vi "-Autonomous Independent.vi"() -> ()   [LabVIEW 2012]
doc: "This VI is called when autonomous begins, and will automatically be terminated when autonomous ends. You can carry out timed or sensor driven robot movement independently without needing to return to the caller."
uses:
  <vilib>/Rock Robotics/WPI/Solenoid/WPI_SolenoidValue.ctl
  Robot Global Data.vi
  <vilib>/Rock Robotics/WPI/RobotDrive/WPI_RobotDriveGetSetRefNum.vi
  <vilib>/addons/control/pid/pid.llb/PID (DBL).vi
  <vilib>/Rock Robotics/WPI/Joystick/WPI_JoystickGetSetRefNum.vi
  <vilib>/Rock Robotics/WPI/Solenoid/WPI_SolenoidSetEnum.vi
  <vilib>/addons/control/pid/NI_PID_pid.lvlib
panel:
  out "Field Position":T1(ring)
  in  "PID gains":T2={"proportional gain (Kc)"=1.0, "integral time (Ti, min)"=0.01, "derivative time (Td, min)"=0.0} {"derivative time (Td, min)" format="%.3f"; "integral time (Ti, min)" format="%.3f"; "proportional gain (Kc)" format="%.3f"}
  in  "Sweet Spot":dbl
  out "tick":dbl
  in  "wait time":dbl
  in  "Fast-Slow Variable":dbl=2.0
  out "Numeric 0":dbl
  out "Current Movement, for debugging":T3 {"Y Joystick Value" scale=1.0..-1.0; "X Joystick Value" scale=-1.0..1.0}
  in  "Array of robot movements":T4(array[cluster]) {"Y Joystick Value" scale=1.0..-1.0; "X Joystick Value" scale=-1.0..1.0}
  # "Be sure to right-click and choose Data Operations>>Make Current Value default if you want to save the array values with the VI"
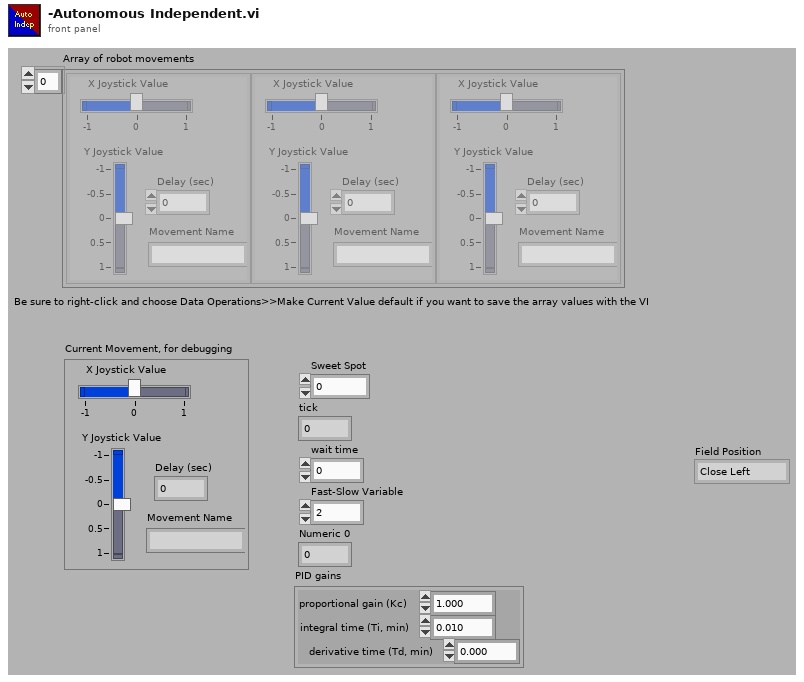
[diagram p1: front panel]
types:
  T1 = enum16{"Close Left", "Close Right", "Far Left", "Far Right"}
  T2 = cluster{"proportional gain (Kc)":dbl, "integral time (Ti, min)":dbl, "derivative time (Td, min)":dbl}
  T3 = cluster{"X Joystick Value":dbl, "Y Joystick Value":dbl, "Delay (sec)":dbl, "Movement Name":string}
  T4 = cluster{"X Joystick Value":dbl, "Y Joystick Value":dbl, "Delay (sec)":dbl, "Movement Name":string}[]
  T5 = typedef "WPI_JoystickDevRef.ctl" = cluster{"Device":T6}
  T6 = typedef "WPI_JoystickDeviceEnum.ctl" = enum16{"USB 1", "USB 2", "USB 3", "USB 4", "Kinect 1", "Kinect 2"}
  T7 = cluster{"axis 1 (x)":dbl, "axis 2 (y)":dbl, "axis 3 (throttle)":dbl, "axis 4":dbl, "axis 5":dbl, "axis 6":dbl}
  T8 = typedef "WPI_SolenoidValue.ctl" = enum16{"Off", "On", "Forward", "Reverse"}
  T9 = typedef "WPI_RobotDriveDevRef.ctl" = cluster{"DevStatus":errorcluster, "Motors[]":T10[], "Square Inputs":bool, "Max Output":dbl, "Isochronous":bool}
  T10 = typedef "WPI_MotorControlDeviceRef.ctl" = cluster{"DeviceStatus":errorcluster, "Type":enum16{"PWM", "CAN"}, "PWM":cluster{"Digital Module":T11, "PWM Channel":T12, "DeadBand":T13}, "CAN":cluster{"Device Number":u8, "Control Mode":T14, "Semaphore":T15, "Max Vout":dbl}, "Invert":bool, "TransformRef":T16, "InvTransformRef":T16}
  T11 = typedef "FPGA_TypedefDigitalModule.ctl" = enum16{"Digital Module 1", "Digital Module 2"}
  T12 = typedef "FPGA_DIOPWMChannel.ctl" = enum8{"PWM 1", "PWM 2", "PWM 3", "PWM 4", "PWM 5", "PWM 6", "PWM 7", "PWM 8", "PWM 9", "PWM 10", "Invalid"}
  T13 = typedef "WPI_PWMDeadband.ctl" = cluster{"Name":string, "maxPositivePwm":i32, "minPositivePwm":i32, "centerPwm":i32, "maxNegativePwm":i32, "minNegativePwm":i32, "angularRange":u16}
  T14 = typedef "WPI_CANJaguar_ControlMode.ctl" = enum8{"Percent VBus", "Current", "Speed", "Position", "Voltage"}
  T15 = typedef "Semaphore RefNum" = refnum<k1>
  T16 = typedef "WPI_PWMTransform_ConPane.ctl" = refnum<vi>
  T17 = cluster{"Center Position":cluster{"X":dbl, "Y":dbl}, "Distance (ft)":dbl, "Center":bool}[]
  T18 = cluster{"Target Info[0]":cluster{"Center Position":cluster{"X":dbl, "Y":dbl}, "Distance (ft)":dbl, "Center":bool}, "Target Info[1]":cluster{"Center Position":cluster{"X":dbl, "Y":dbl}, "Distance (ft)":dbl, "Center":bool}, "Target Info[2]":cluster{"Center Position":cluster{"X":dbl, "Y":dbl}, "Distance (ft)":dbl, "Center":bool}, "Target Info[3]":cluster{"Center Position":cluster{"X":dbl, "Y":dbl}, "Distance (ft)":dbl, "Center":bool}, "Target Info[4]":cluster{"Center Position":cluster{"X":dbl, "Y":dbl}, "Distance (ft)":dbl, "Center":bool}, "Target Info[5]":cluster{"Center Position":cluster{"X":dbl, "Y":dbl}, "Distance (ft)":dbl, "Center":bool}, "Target Info[6]":cluster{"Center Position":cluster{"X":dbl, "Y":dbl}, "Distance (ft)":dbl, "Center":bool}, "Target Info[7]":cluster{"Center Position":cluster{"X":dbl, "Y":dbl}, "Distance (ft)":dbl, "Center":bool}, "Target Info[8]":cluster{"Center Position":cluster{"X":dbl, "Y":dbl}, "Distance (ft)":dbl, "Center":bool}}
  T19 = cluster{"Center Position":cluster{"X":dbl, "Y":dbl}, "Distance (ft)":dbl, "Center":bool}
  T20 = typedef "WPI_SolenoidDevRef.ctl" = cluster{"DevStatus":errorcluster, "Solenoid Module":T21, "Forward Solenoid Channel":T22, "Reverse Solenoid Channel":T22}
  T21 = typedef "FPGA_TypedefSolenoidModule.ctl" = enum16{"Solenoid Module 1", "Solenoid Module 2"}
  T22 = typedef "WPI_SolenoidChannel.ctl" = enum8{"Solenoid 1", "Solenoid 2", "Solenoid 3", "Solenoid 4", "Solenoid 5", "Solenoid 6", "Solenoid 7", "Solenoid 8", "Invalid"}
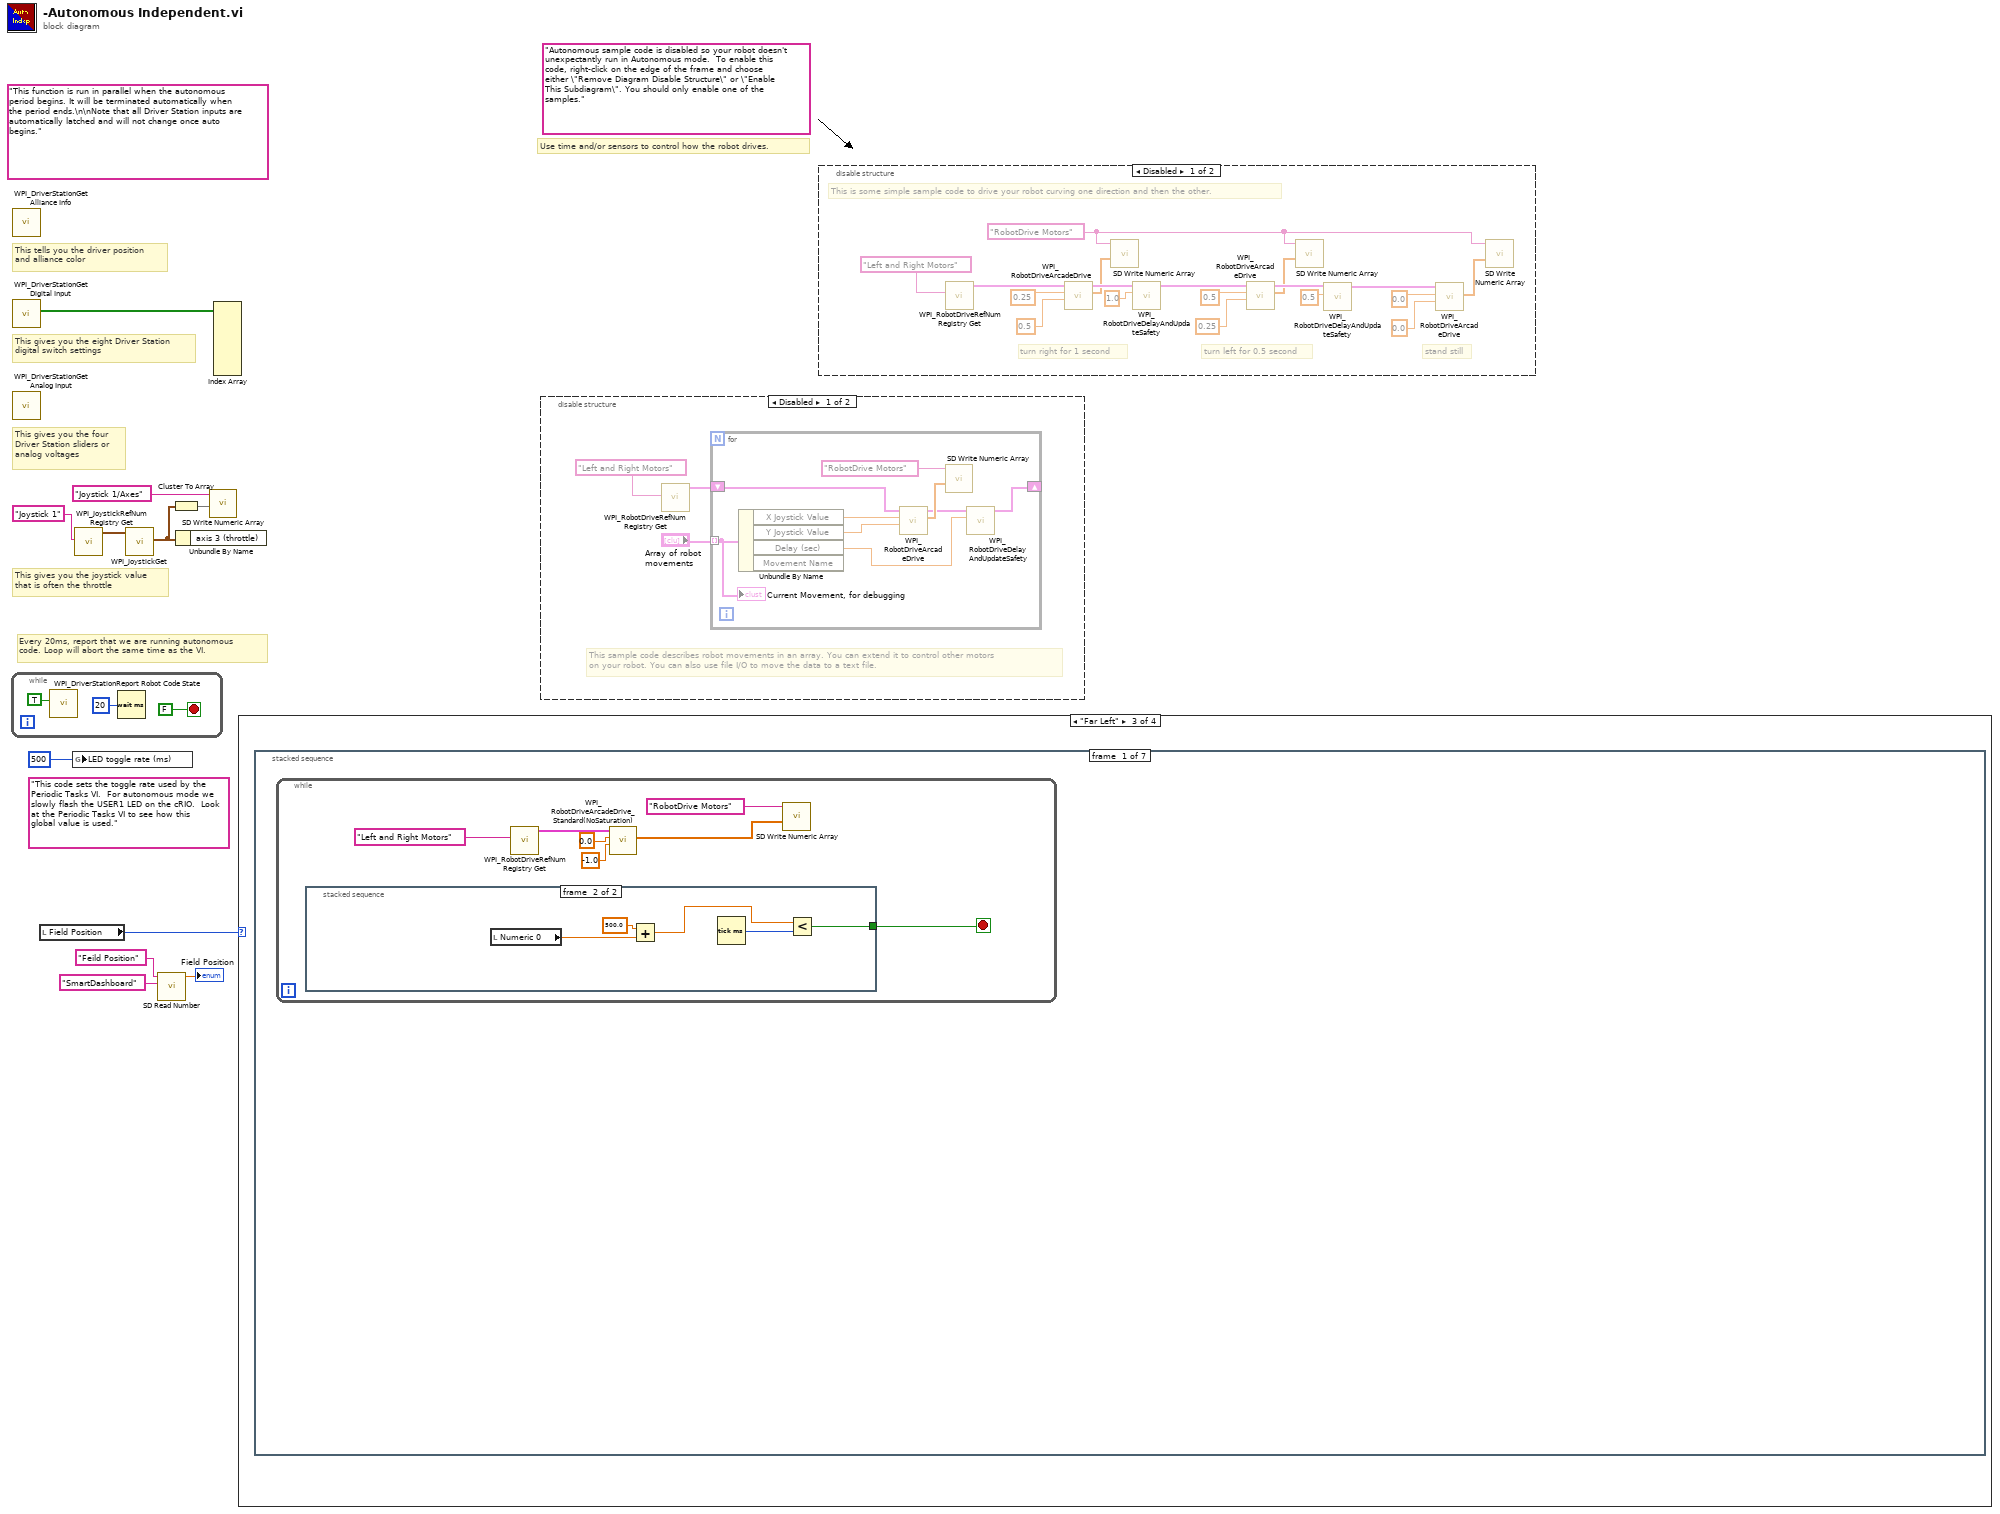
[diagram p0: block diagram]
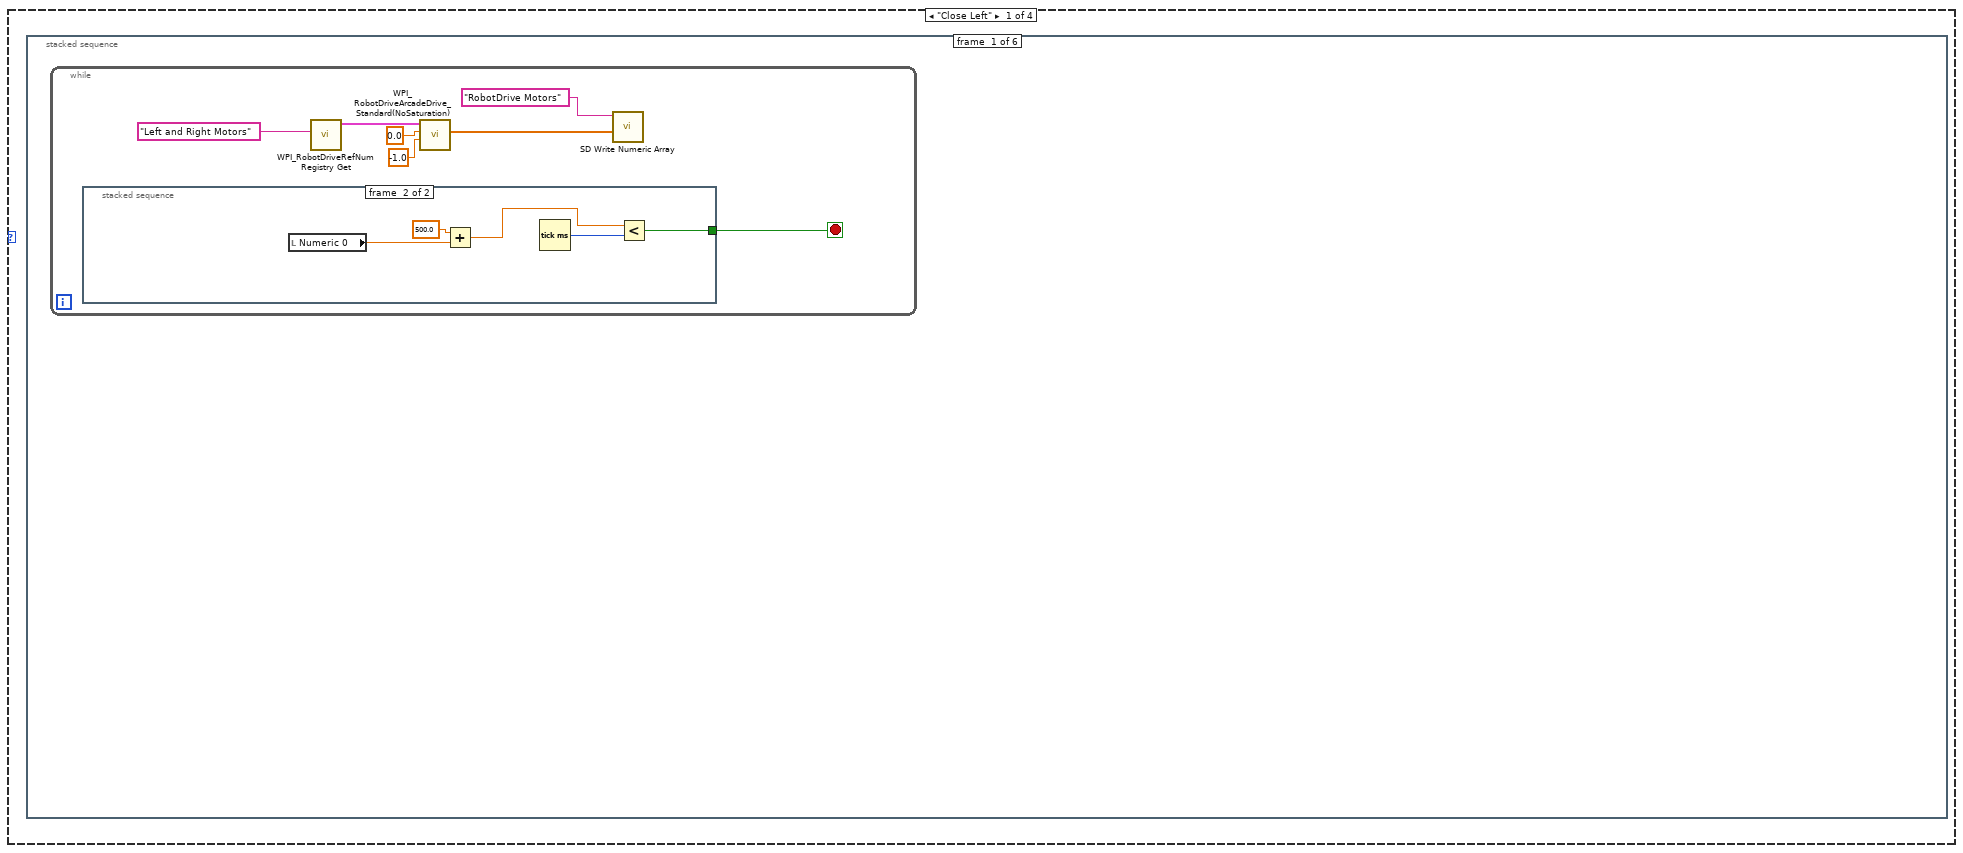
[diagram p2: hidden frame]
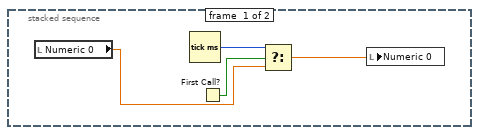
[diagram p3: hidden frame]
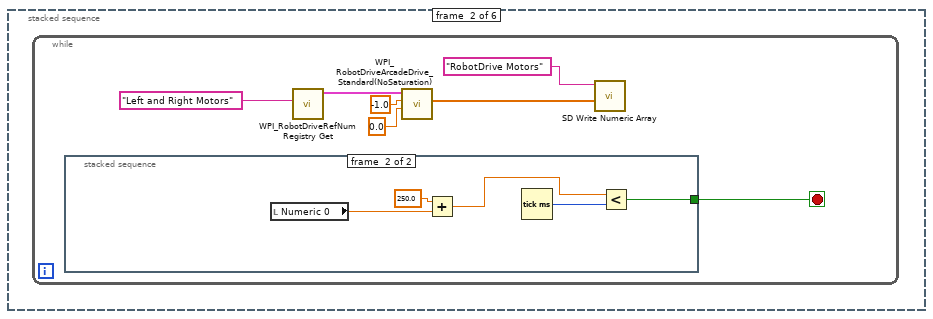
[diagram p4: hidden frame]
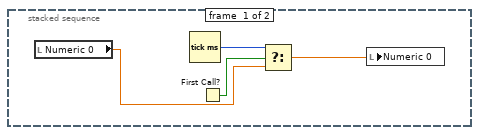
[diagram p5: hidden frame]
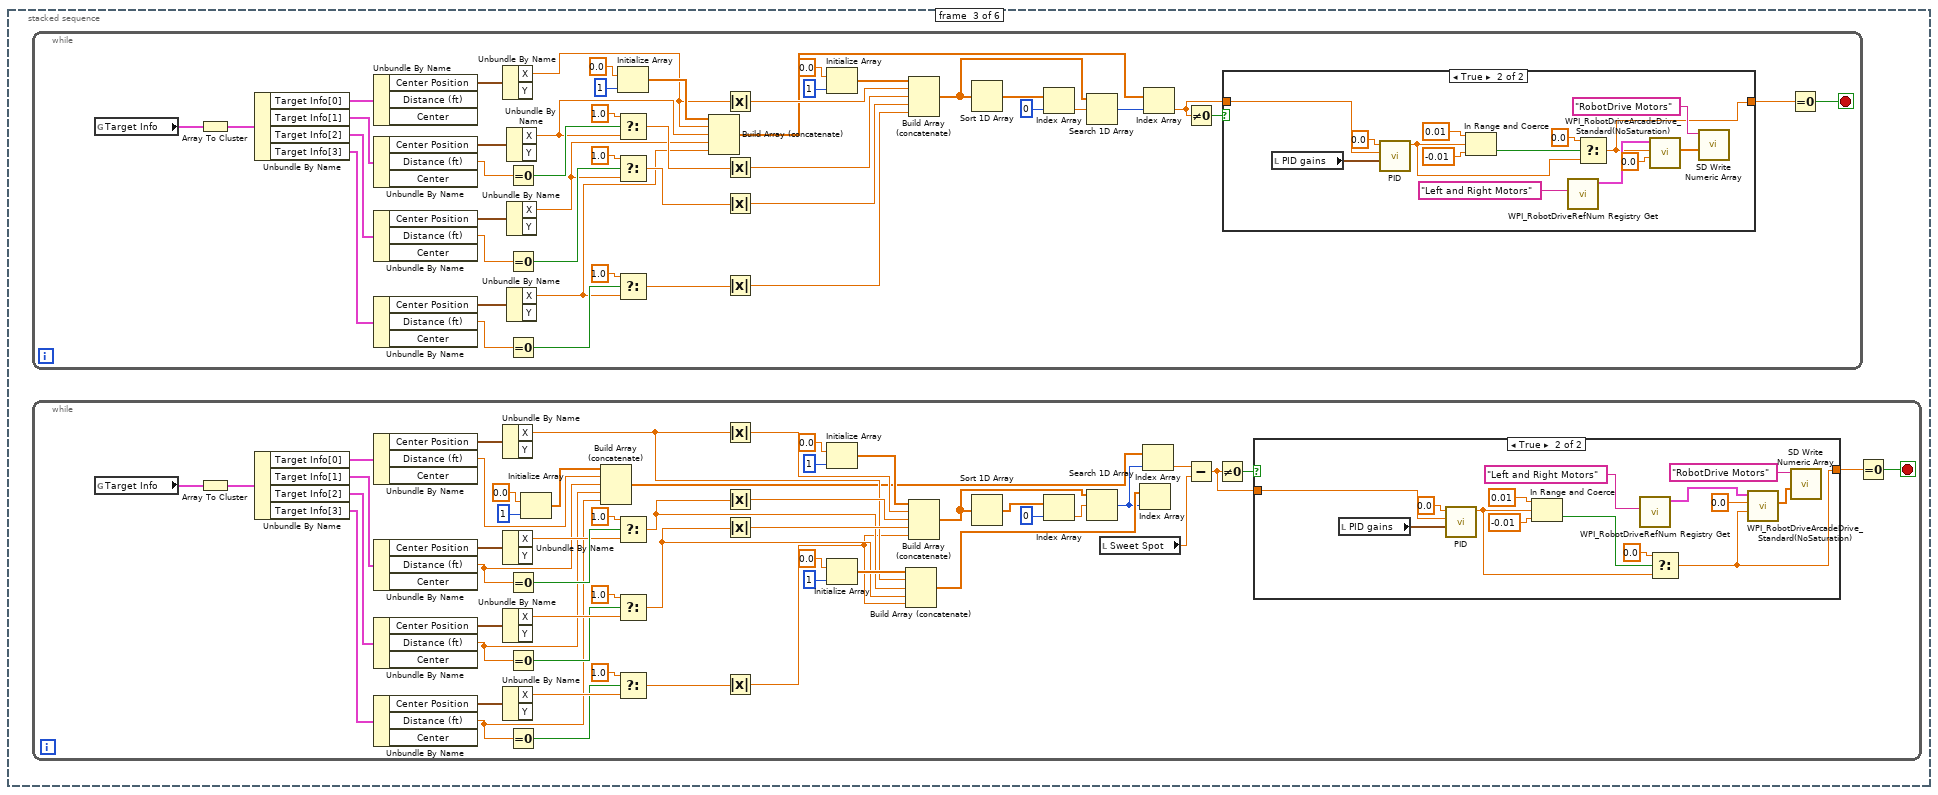
[diagram p6: hidden frame]
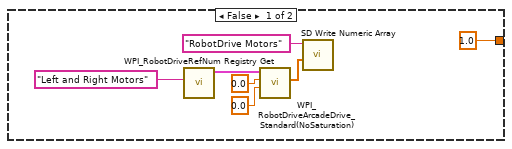
[diagram p7: hidden frame]
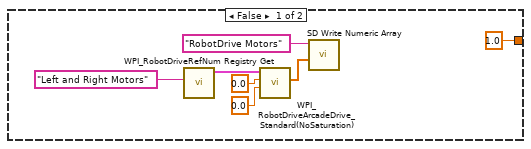
[diagram p8: hidden frame]
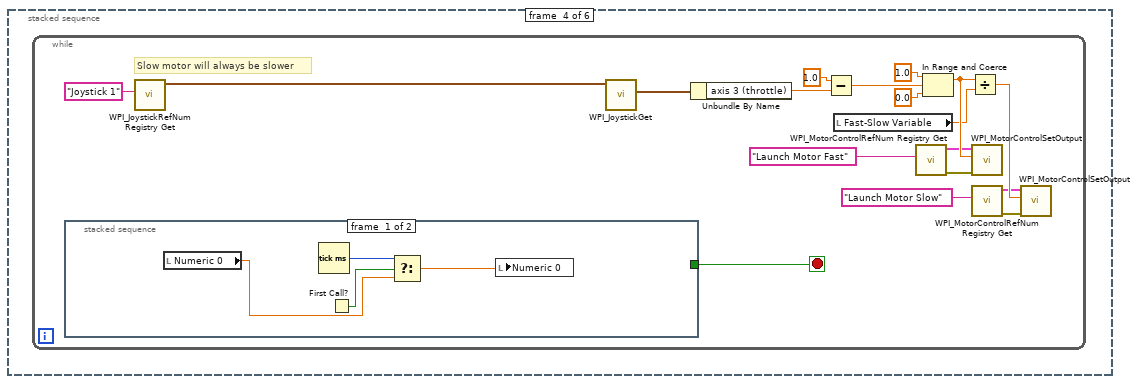
[diagram p9: hidden frame]
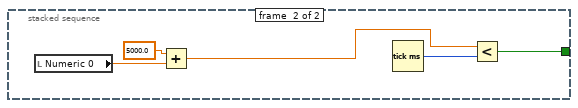
[diagram p10: hidden frame]
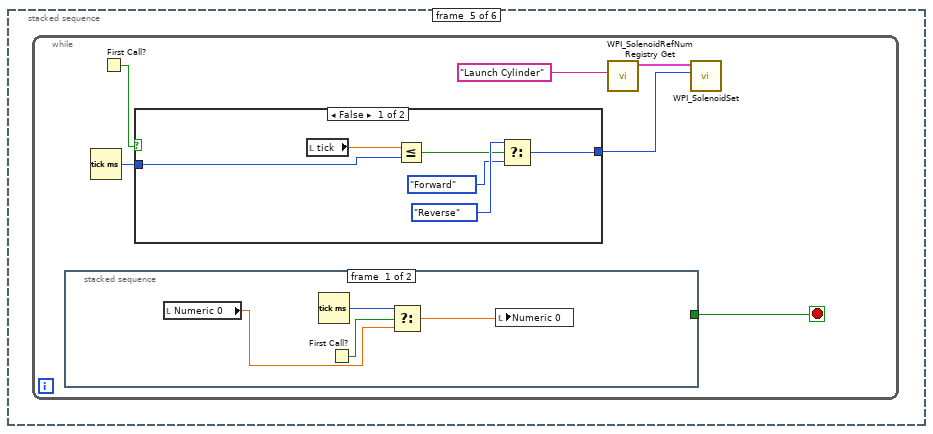
[diagram p11: hidden frame]
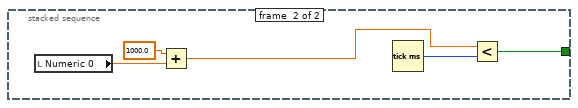
[diagram p12: hidden frame]
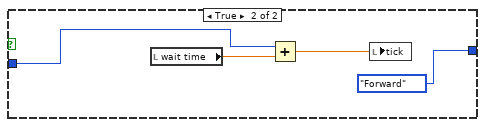
[diagram p13: hidden frame]
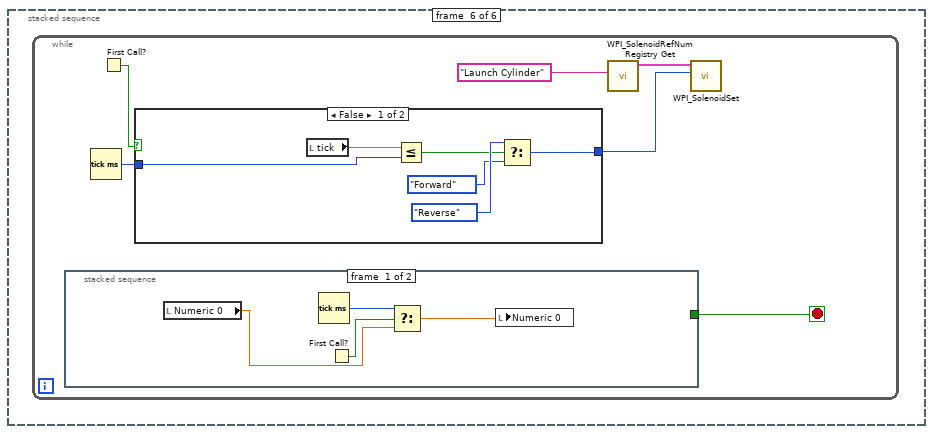
[diagram p14: hidden frame]
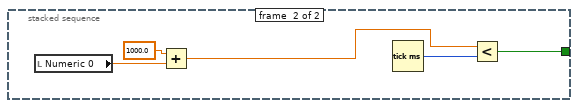
[diagram p15: hidden frame]
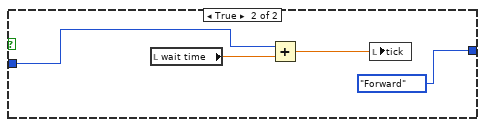
[diagram p16: hidden frame]
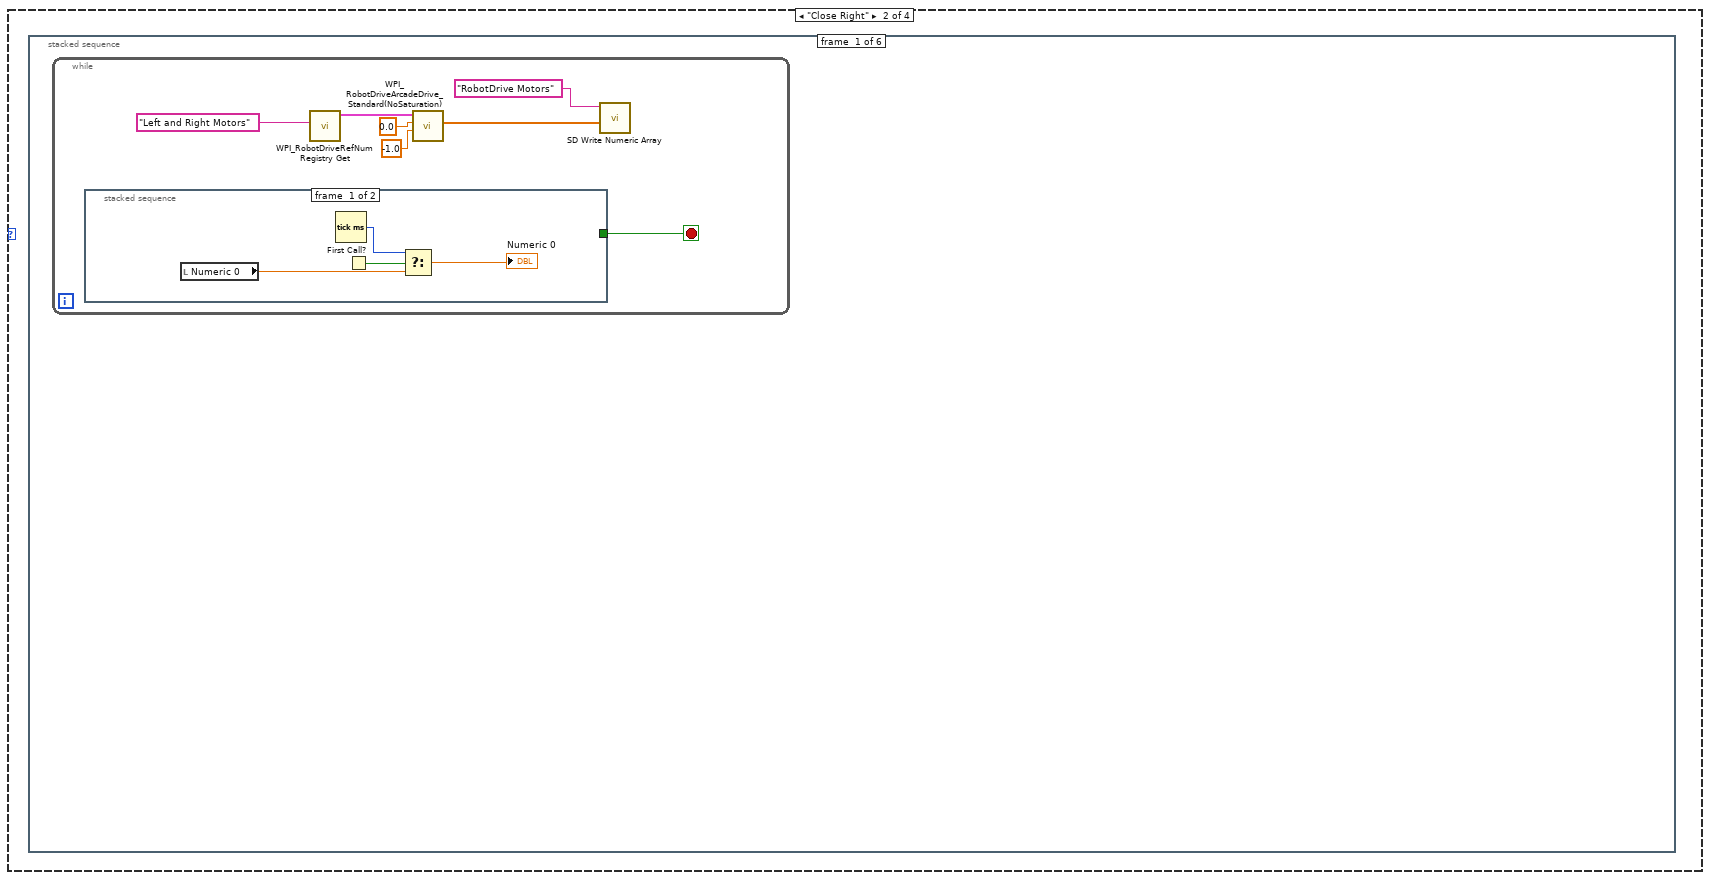
[diagram p17: hidden frame]
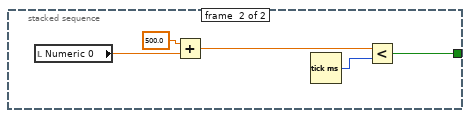
[diagram p18: hidden frame]
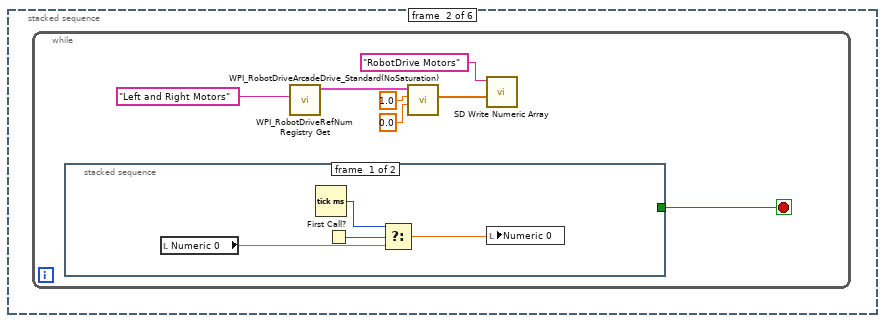
[diagram p19: hidden frame]
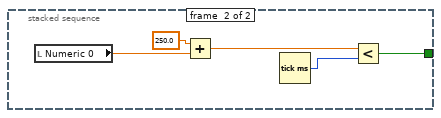
[diagram p20: hidden frame]
diagram:
  (unwired) "This code sets the toggle rate used by the Periodic Tasks VI.  For autonomous mode we slowly flash the USER1 LED on the cRIO.  Look at the Periodic Tasks VI to see how this global value is used."
  (unwired) "Autonomous sample code is disabled so your robot doesn't unexpectantly run in Autonomous mode.  To enable this code, right-click on the edge of the frame and choose either \"Remove Diagram Disable Structure\" or \"Enable This Subdiagram\". You should only enable one of the samples."
  (unwired) "This function is run in parallel when the autonomous period begins. It will be terminated automatically when the period ends.\n\nNote that all Driver Station inputs are automatically latched and will not change once auto begins."
  # "Every 20ms, report that we are running autonomous\ncode. Loop will abort the same time as the VI."
  # "This gives you the joystick value\nthat is often the throttle"
  # "Use time and/or sensors to control how the robot drives."
  # "This tells you the driver position\nand alliance color"
  # "This gives you the eight Driver Station\ndigital switch settings"
  # "This gives you the four\nDriver Station sliders or\nanalog voltages"
  n1 = while {
    stop <- FALSE stop-if-true
    n2 = call <vilib>:"WPI_DriverStationReport Robot Code State.vi"("Autonomous"=TRUE) -> ()  [unwired: 10 in, 1 out]
    n3 = Wait (ms)(milliseconds to wait=u32 20) -> ()  [unwired: 1 out]
  }
  n4 = call <vilib>:"WPI_DriverStationGet Alliance Info.vi"() -> ()  [unwired: 12 out]
  n5 = call <vilib>:"WPI_DriverStationGet Digital Input.vi"() -> ("Driver Station Digital Input (1-8)"=w11:bool[])  [unwired: 11 out]
  n6 = call <vilib>:"WPI_DriverStationGet Analog Input.vi"() -> ()  [unwired: 12 out]
  n7 = local read "Field Position"() -> (w1:T1)
  n8 = global write "Robot Global Data.vi" "LED toggle rate (ms)"(u32 500 ("LED ms toggle rate")) -> ()
  n9 = call <vilib>:"WPI_JoystickRefNum Registry Get.vi"("refnum name"="Joystick 1") -> ("JoystickDevRef"=w9:T5)  [unwired: 1 in, 9 out]
  n10 = call <vilib>:"WPI_JoystickGet.vi"("JoystickDevRef"=w9) -> ("Axes"=w6:T7)  [unwired: 1 in, 5 out]
  n11 = call <vilib>:"SD Read Number.vi"("Table Prefix"="SmartDashboard", "Name"="Feild Position") -> ("Numeric"=→"Field Position":dbl)  [unwired: 7 in, 2 out]
  n12 = Cluster To Array(cluster=w6) -> (array=w7:dbl[])
  n13 = Unbundle By Name(w6) -> ()  [unwired: 1 out]
  n14 = call <vilib>:"SD Write Numeric Array.vi"("Numeric Array"=w7, "Name"="Joystick 1/Axes") -> ()  [unwired: 8 in, 2 out]
  n15 = Index Array(array=w11) -> ()  [unwired: 8 in, 8 out]
  n16 = case shown="\"Far Left\"" w1 {
    frame "Close Left" {
      n17 = stacked-sequence {
        frame #0 {
          n18 = while {
            stop <- w15 stop-if-true
            n19 = stacked-sequence {
              tunnel: [_ w26] -> w15
              frame #0 {
                n20 = local read "Numeric 0"() -> (w23:dbl)
                n21 = Tick Count (ms)() -> (millisecond timer value=w24:u32)
                n22 = First Call?() -> (First Call?: T/F=w25:bool)
                n23 = Select(t=w24, s=w25, f=w23) -> (s? t:f=w22:dbl)
                n24 = local write "Numeric 0"(w22) -> ()
              }
              frame #1 {
                n25 = local read "Numeric 0"() -> (w29:dbl)
                n26 = Add(x=500.0, y=w29) -> (x+y=w28:dbl)
                n27 = Tick Count (ms)() -> (millisecond timer value=w27:u32)
                n28 = Less?(x=w28, y=w27) -> (x < y?=w26:bool)
              }
            }
            n29 = call <vilib>:"WPI_RobotDriveRefNum Registry Get.vi"("refnum name"="Left and Right Motors") -> ("RobotDriveDevRef"=w20:T9)  [unwired: 1 in, 9 out]
            n30 = call <vilib>:"WPI_RobotDriveArcadeDrive_Standard(NoSaturation).vi"("Y axis value"=-1.0 ("X axis value"), "X axis value"=0.0, "RobotDriveDevRef"=w20) -> ("Motor Values"=w18:dbl[])  [unwired: 1 in, 7 out]
            n31 = call <vilib>:"SD Write Numeric Array.vi"("Numeric Array"=w18, "Name"="RobotDrive Motors") -> ()  [unwired: 8 in, 2 out]
          }
        }
        frame #1 {
          n32 = while {
            stop <- w31 stop-if-true
            n33 = stacked-sequence {
              tunnel: [_ w42] -> w31
              frame #0 {
                n34 = local read "Numeric 0"() -> (w39:dbl)
                n35 = Tick Count (ms)() -> (millisecond timer value=w40:u32)
                n36 = First Call?() -> (First Call?: T/F=w41:bool)
                n37 = Select(t=w40, s=w41, f=w39) -> (s? t:f=w38:dbl)
                n38 = local write "Numeric 0"(w38) -> ()
              }
              frame #1 {
                n39 = local read "Numeric 0"() -> (w45:dbl)
                n40 = Add(x=250.0, y=w45) -> (x+y=w44:dbl)
                n41 = Tick Count (ms)() -> (millisecond timer value=w43:u32)
                n42 = Less?(x=w44, y=w43) -> (x < y?=w42:bool)
              }
            }
            n43 = call <vilib>:"WPI_RobotDriveRefNum Registry Get.vi"("refnum name"="Left and Right Motors") -> ("RobotDriveDevRef"=w33:T9)  [unwired: 1 in, 9 out]
            n44 = call <vilib>:"WPI_RobotDriveArcadeDrive_Standard(NoSaturation).vi"("Y axis value"=0.0 ("X axis value"), "X axis value"=-1.0, "RobotDriveDevRef"=w33) -> ("Motor Values"=w35:dbl[])  [unwired: 1 in, 7 out]
            n45 = call <vilib>:"SD Write Numeric Array.vi"("Numeric Array"=w35, "Name"="RobotDrive Motors") -> ()  [unwired: 8 in, 2 out]
          }
        }
        frame #2 {
          n46 = while {
            stop <- w74 stop-if-true
            n47 = global read "Robot Global Data.vi" "Target Info"() -> (w92:T17)
            n48 = Array To Cluster(array=w92) -> (cluster=w91:T18)
            n49 = Unbundle By Name(w91) -> ("Target Info[0]"=w90:T19, "Target Info[1]"=w85:T19, "Target Info[2]"=w84:T19, "Target Info[3]"=w83:T19)
            n50 = Unbundle By Name(w90) -> ("Center Position"=w89:cluster{"X":dbl, "Y":dbl})  [unwired: 2 out]
            n51 = Unbundle By Name(w85) -> ("Center Position"=w88:cluster{"X":dbl, "Y":dbl}, "Distance (ft)"=w51:dbl)  [unwired: 1 out]
            n52 = Unbundle By Name(w84) -> ("Center Position"=w87:cluster{"X":dbl, "Y":dbl}, "Distance (ft)"=w53:dbl)  [unwired: 1 out]
            n53 = Unbundle By Name(w83) -> ("Center Position"=w86:cluster{"X":dbl, "Y":dbl}, "Distance (ft)"=w55:dbl)  [unwired: 1 out]
            n54 = Unbundle By Name(w89) -> ("X"=w49:dbl)  [unwired: 1 out]
            n55 = Unbundle By Name(w88) -> ("X"=w50:dbl)  [unwired: 1 out]
            n56 = Unbundle By Name(w87) -> ("X"=w52:dbl)  [unwired: 1 out]
            n57 = Unbundle By Name(w86) -> ("X"=w54:dbl)  [unwired: 1 out]
            n58 = Equal To 0?(x=w51) -> (x = 0?=w82:bool)
            n59 = Equal To 0?(x=w53) -> (x = 0?=w81:bool)
            n60 = Equal To 0?(x=w55) -> (x = 0?=w80:bool)
            n61 = Initialize Array(0.0 ("element"), 1 ("dimension size")) -> (w58:dbl[])
            n62 = Select(t=1.0, s=w82, f=w50) -> (s? t:f=w63:dbl)
            n63 = Select(t=1.0, s=w81, f=w52) -> (s? t:f=w62:dbl)
            n64 = Select(t=1.0, s=w80, f=w54) -> (s? t:f=w76:dbl)
            n65 = Build Array (concatenate)(w58, w49, w50, w52, w54) -> (w57:dbl[])
            n66 = Absolute Value(x=w49) -> (abs(x)=w70:dbl)
            n67 = Absolute Value(x=w63) -> (abs(x)=w69:dbl)
            n68 = Absolute Value(x=w62) -> (abs(x)=w68:dbl)
            n69 = Absolute Value(x=w76) -> (abs(x)=w61:dbl)
            n70 = Initialize Array(0.0 ("element"), 1 ("dimension size")) -> (w71:dbl[])
            n71 = Build Array (concatenate)(w71, w70, w69, w68, w61) -> (w64:dbl[])
            n72 = Sort 1D Array(array=w64) -> (sorted array=w67:dbl[])
            n73 = Index Array(array=w67, index=0) -> (element=w65:dbl)
            n74 = Search 1D Array(1D array=w64, element=w65) -> (index of element=w56:i32)  [unwired: 1 in]
            n75 = Index Array(array=w57, index=w56) -> (element=w47:dbl)
            n76 = Not Equal To 0?(x=w47) -> (x != 0?=w48:bool)
            n77 = case shown="True" w48 {
              tunnel: [1.0 ("output") w102] -> w75
              tunnel: w47 -> [_ w101]
              frame False {
                n78 = call <vilib>:"WPI_RobotDriveRefNum Registry Get.vi"("refnum name"="Left and Right Motors") -> ("RobotDriveDevRef"=w98:T9)  [unwired: 1 in, 9 out]
                n79 = call <vilib>:"WPI_RobotDriveArcadeDrive_Standard(NoSaturation).vi"("Y axis value"=0.0, "X axis value"=0.0, "RobotDriveDevRef"=w98) -> ("Motor Values"=w96:dbl[])  [unwired: 1 in, 7 out]
                n80 = call <vilib>:"SD Write Numeric Array.vi"("Numeric Array"=w96, "Name"="RobotDrive Motors") -> ()  [unwired: 8 in, 2 out]
              }
              frame True {
                n81 = local read "PID gains"() -> (w100:T2)
                n82 = call-poly <vilib>:"PID.vi"("PID gains"=w100, "process variable"=w101, "setpoint"=0.0 ("process variable")) -> ("output"=w103:dbl)  [unwired: 7 in, 1 out]
                n83 = In Range and Coerce(upper limit=0.01, x=w103, lower limit=-0.01) -> (In Range?=w105:bool)  [unwired: 1 out]
                n84 = call <vilib>:"WPI_RobotDriveRefNum Registry Get.vi"("refnum name"="Left and Right Motors") -> ("RobotDriveDevRef"=w111:T9)  [unwired: 1 in, 9 out]
                n85 = Select(t=0.0, s=w105, f=w103) -> (s? t:f=w102:dbl)
                n86 = call <vilib>:"WPI_RobotDriveArcadeDrive_Standard(NoSaturation).vi"("Y axis value"=0.0, "X axis value"=w102, "RobotDriveDevRef"=w111) -> ("Motor Values"=w110:dbl[])  [unwired: 1 in, 7 out]
                n87 = call <vilib>:"SD Write Numeric Array.vi"("Numeric Array"=w110, "Name"="RobotDrive Motors") -> ()  [unwired: 8 in, 2 out]
              }
            }
            n88 = Equal To 0?(x=w75) -> (x = 0?=w74:bool)
          }
          n89 = while {
            stop <- w145 stop-if-true
            n90 = global read "Robot Global Data.vi" "Target Info"() -> (w166:T17)
            n91 = Array To Cluster(array=w166) -> (cluster=w165:T18)
            n92 = Unbundle By Name(w165) -> ("Target Info[0]"=w164:T19, "Target Info[1]"=w159:T19, "Target Info[2]"=w158:T19, "Target Info[3]"=w157:T19)
            n93 = Unbundle By Name(w164) -> ("Center Position"=w163:cluster{"X":dbl, "Y":dbl}, "Distance (ft)"=w123:dbl)  [unwired: 1 out]
            n94 = Unbundle By Name(w159) -> ("Center Position"=w162:cluster{"X":dbl, "Y":dbl}, "Distance (ft)"=w122:dbl)  [unwired: 1 out]
            n95 = Unbundle By Name(w158) -> ("Center Position"=w161:cluster{"X":dbl, "Y":dbl}, "Distance (ft)"=w121:dbl)  [unwired: 1 out]
            n96 = Unbundle By Name(w157) -> ("Center Position"=w160:cluster{"X":dbl, "Y":dbl}, "Distance (ft)"=w120:dbl)  [unwired: 1 out]
            n97 = Unbundle By Name(w163) -> ("X"=w131:dbl)  [unwired: 1 out]
            n98 = Unbundle By Name(w162) -> ("X"=w148:dbl)  [unwired: 1 out]
            n99 = Unbundle By Name(w161) -> ("X"=w155:dbl)  [unwired: 1 out]
            n100 = Unbundle By Name(w160) -> ("X"=w156:dbl)  [unwired: 1 out]
            n101 = Equal To 0?(x=w122) -> (x = 0?=w154:bool)
            n102 = Equal To 0?(x=w121) -> (x = 0?=w153:bool)
            n103 = Equal To 0?(x=w120) -> (x = 0?=w152:bool)
            n104 = Initialize Array(0.0 ("element"), 1 ("dimension size")) -> (w124:dbl[])
            n105 = Build Array (concatenate)(w124, w123, w122, w121, w120) -> (w119:dbl[])
            n106 = Select(t=1.0, s=w154, f=w148) -> (s? t:f=w130:dbl)
            n107 = Select(t=1.0, s=w153, f=w155) -> (s? t:f=w129:dbl)
            n108 = Select(t=1.0, s=w152, f=w156) -> (s? t:f=w147:dbl)
            n109 = Absolute Value(x=w131) -> (abs(x)=w141:dbl)
            n110 = Absolute Value(x=w130) -> (abs(x)=w140:dbl)
            n111 = Absolute Value(x=w129) -> (abs(x)=w139:dbl)
            n112 = Absolute Value(x=w147) -> (abs(x)=w128:dbl)
            n113 = Initialize Array(0.0 ("element"), 1 ("dimension size")) -> (w142:dbl[])
            n114 = Initialize Array(0.0 ("element"), 1 ("dimension size")) -> (w132:dbl[])
            n115 = Build Array (concatenate)(w132, w131, w130, w129, w128) -> (w127:dbl[])
            n116 = Build Array (concatenate)(w142, w141, w140, w139, w128) -> (w135:dbl[])
            n117 = Sort 1D Array(array=w135) -> (sorted array=w138:dbl[])
            n118 = Index Array(array=w138, index=0) -> (element=w136:dbl)
            n119 = Search 1D Array(1D array=w135, element=w136) -> (index of element=w118:i32)  [unwired: 1 in]
            n120 = local read "Sweet Spot"() -> (w114:dbl)
            n121 = Index Array(array=w127, index=w118) -> ()  [unwired: 1 out]
            n122 = Index Array(array=w119, index=w118) -> (element=w117:dbl)
            n123 = Subtract(x=w117, y=w114) -> (x-y=w116:dbl)
            n124 = Not Equal To 0?(x=w116) -> (x != 0?=w115:bool)
            n125 = case shown="True" w115 {
              tunnel: [1.0 ("output") w176] -> w146
              tunnel: w116 -> [_ w177]
              frame False {
                n126 = call <vilib>:"WPI_RobotDriveRefNum Registry Get.vi"("refnum name"="Left and Right Motors") -> ("RobotDriveDevRef"=w172:T9)  [unwired: 1 in, 9 out]
                n127 = call <vilib>:"WPI_RobotDriveArcadeDrive_Standard(NoSaturation).vi"("Y axis value"=0.0, "X axis value"=0.0, "RobotDriveDevRef"=w172) -> ("Motor Values"=w170:dbl[])  [unwired: 1 in, 7 out]
                n128 = call <vilib>:"SD Write Numeric Array.vi"("Numeric Array"=w170, "Name"="RobotDrive Motors") -> ()  [unwired: 8 in, 2 out]
              }
              frame True {
                n129 = local read "PID gains"() -> (w174:T2)
                n130 = call-poly <vilib>:"PID.vi"("PID gains"=w174, "process variable"=w177, "setpoint"=0.0 ("process variable")) -> ("output"=w178:dbl)  [unwired: 7 in, 1 out]
                n131 = In Range and Coerce(upper limit=0.01, x=w178, lower limit=-0.01) -> (In Range?=w180:bool)  [unwired: 1 out]
                n132 = call <vilib>:"WPI_RobotDriveRefNum Registry Get.vi"("refnum name"="Left and Right Motors") -> ("RobotDriveDevRef"=w185:T9)  [unwired: 1 in, 9 out]
                n133 = Select(t=0.0, s=w180, f=w178) -> (s? t:f=w176:dbl)
                n134 = call <vilib>:"WPI_RobotDriveArcadeDrive_Standard(NoSaturation).vi"("Y axis value"=w176, "X axis value"=0.0, "RobotDriveDevRef"=w185) -> ("Motor Values"=w184:dbl[])  [unwired: 1 in, 7 out]
                n135 = call <vilib>:"SD Write Numeric Array.vi"("Numeric Array"=w184, "Name"="RobotDrive Motors") -> ()  [unwired: 8 in, 2 out]
              }
            }
            n136 = Equal To 0?(x=w146) -> (x = 0?=w145:bool)
          }
        }
        frame #3 {
          n137 = while {
            stop <- w189 stop-if-true
            # "Slow motor will always be slower"
            n138 = stacked-sequence {
              tunnel: [_ w210] -> w189
              frame #0 {
                n139 = local read "Numeric 0"() -> (w207:dbl)
                n140 = Tick Count (ms)() -> (millisecond timer value=w208:u32)
                n141 = First Call?() -> (First Call?: T/F=w209:bool)
                n142 = Select(t=w208, s=w209, f=w207) -> (s? t:f=w206:dbl)
                n143 = local write "Numeric 0"(w206) -> ()
              }
              frame #1 {
                n144 = local read "Numeric 0"() -> (w213:dbl)
                n145 = Add(x=5000.0, y=w213) -> (x+y=w212:dbl)
                n146 = Tick Count (ms)() -> (millisecond timer value=w211:u32)
                n147 = Less?(x=w212, y=w211) -> (x < y?=w210:bool)
              }
            }
            n148 = call <vilib>:"WPI_JoystickRefNum Registry Get.vi"("refnum name"="Joystick 1") -> ("JoystickDevRef"=w203:T5)  [unwired: 1 in, 9 out]
            n149 = call <vilib>:"WPI_JoystickGet.vi"("JoystickDevRef"=w203) -> ("Axes"=w204:T7)  [unwired: 1 in, 5 out]
            n150 = Unbundle By Name(w204) -> ("axis 3 (throttle)"=w205:dbl)
            n151 = Subtract(x=1.0, y=w205) -> (x-y=w199:dbl)
            n152 = local read "Fast-Slow Variable"() -> (w188:dbl)
            n153 = call <vilib>:"WPI_MotorControlRefNum Registry Get.vi"("refnum name"="Launch Motor Fast") -> ("error out"=w194:errorcluster, "MotorControlDevRef"=w193:T10)  [unwired: 9 in]
            n154 = In Range and Coerce(upper limit=1.0, x=w199, lower limit=0.0) -> (coerced(x)=w198:dbl)  [unwired: 1 out]
            n155 = Divide(x=w198, y=w188) -> (x/y=w196:dbl)
            n156 = call <vilib>:"WPI_MotorControlSetOutput.vi"("error in (no error)"=w194, "Output"=w198, "MotorControlDevRef"=w193) -> ()  [unwired: 6 in, 3 out]
            n157 = call <vilib>:"WPI_MotorControlRefNum Registry Get.vi"("refnum name"="Launch Motor Slow") -> ("error out"=w191:errorcluster, "MotorControlDevRef"=w192:T10)  [unwired: 9 in]
            n158 = call <vilib>:"WPI_MotorControlSetOutput.vi"("error in (no error)"=w191, "Output"=w196, "MotorControlDevRef"=w192) -> ()  [unwired: 6 in, 3 out]
          }
        }
        frame #4 {
          n159 = while {
            stop <- w215 stop-if-true
            n160 = stacked-sequence {
              tunnel: [_ w225] -> w215
              frame #0 {
                n161 = local read "Numeric 0"() -> (w222:dbl)
                n162 = Tick Count (ms)() -> (millisecond timer value=w223:u32)
                n163 = First Call?() -> (First Call?: T/F=w224:bool)
                n164 = Select(t=w223, s=w224, f=w222) -> (s? t:f=w221:dbl)
                n165 = local write "Numeric 0"(w221) -> ()
              }
              frame #1 {
                n166 = local read "Numeric 0"() -> (w228:dbl)
                n167 = Add(x=1000.0, y=w228) -> (x+y=w227:dbl)
                n168 = Tick Count (ms)() -> (millisecond timer value=w226:u32)
                n169 = Less?(x=w227, y=w226) -> (x < y?=w225:bool)
              }
            }
            n170 = Tick Count (ms)() -> (millisecond timer value=w216:u32)
            n171 = First Call?() -> (First Call?: T/F=w220:bool)
            n172 = case shown="False" w220 {
              tunnel: w216 -> [w234 w239]
              tunnel: [w230 WPI_SolenoidValue."Forward" ("Value")] -> w219
              frame False {
                n173 = local read "tick"() -> (w235:dbl)
                n174 = Less Or Equal?(x=w235, y=w234) -> (x <= y?=w231:bool)
                n175 = Select(t=WPI_SolenoidValue."Reverse" ("Value"), s=w231, f=WPI_SolenoidValue."Forward" ("Value")) -> (s? t:f=w230:T8)
              }
              frame True {
                n176 = local read "wait time"() -> (w236:dbl)
                n177 = Add(x=w239, y=w236) -> (x+y=w237:dbl)
                n178 = local write "tick"(w237) -> ()
              }
            }
            n179 = call <vilib>:"WPI_SolenoidRefNum Registry Get.vi"("refnum name"="Launch Cylinder") -> ("SolenoidDevRef"=w218:T20)  [unwired: 9 in, 1 out]
            n180 = call-poly <vilib>:"WPI_SolenoidSet.vi"("Value"=w219, "SolenoidDevRef"=w218) -> ()  [unwired: 8 in, 2 out]
          }
        }
        frame #5 {
          n181 = while {
            stop <- w240 stop-if-true
            n182 = stacked-sequence {
              tunnel: [_ w251] -> w240
              frame #0 {
                n183 = local read "Numeric 0"() -> (w247:dbl)
                n184 = Tick Count (ms)() -> (millisecond timer value=w248:u32)
                n185 = First Call?() -> (First Call?: T/F=w249:bool)
                n186 = Select(t=w248, s=w249, f=w247) -> (s? t:f=w246:dbl)
                n187 = local write "Numeric 0"(w246) -> ()
              }
              frame #1 {
                n188 = local read "Numeric 0"() -> (w250:dbl)
                n189 = Add(x=1000.0, y=w250) -> (x+y=w253:dbl)
                n190 = Tick Count (ms)() -> (millisecond timer value=w252:u32)
                n191 = Less?(x=w253, y=w252) -> (x < y?=w251:bool)
              }
            }
            n192 = Tick Count (ms)() -> (millisecond timer value=w241:u32)
            n193 = First Call?() -> (First Call?: T/F=w245:bool)
            n194 = case shown="False" w245 {
              tunnel: w241 -> [w260 w264]
              tunnel: [w256 WPI_SolenoidValue."Forward" ("Value")] -> w244
              frame False {
                n195 = local read "tick"() -> (w255:dbl)
                n196 = Less Or Equal?(x=w255, y=w260) -> (x <= y?=w257:bool)
                n197 = Select(t=WPI_SolenoidValue."Reverse" ("Value"), s=w257, f=WPI_SolenoidValue."Forward" ("Value")) -> (s? t:f=w256:T8)
              }
              frame True {
                n198 = local read "wait time"() -> (w262:dbl)
                n199 = Add(x=w264, y=w262) -> (x+y=w261:dbl)
                n200 = local write "tick"(w261) -> ()
              }
            }
            n201 = call <vilib>:"WPI_SolenoidRefNum Registry Get.vi"("refnum name"="Launch Cylinder") -> ("SolenoidDevRef"=w243:T20)  [unwired: 9 in, 1 out]
            n202 = call-poly <vilib>:"WPI_SolenoidSet.vi"("Value"=w244, "SolenoidDevRef"=w243) -> ()  [unwired: 8 in, 2 out]
          }
        }
      }
    }
    frame "Close Right" {
      n203 = stacked-sequence {
        frame #0 {
          n204 = while {
            stop <- w265 stop-if-true
            n205 = stacked-sequence {
              tunnel: [_ w276] -> w265
              frame #0 {
                n206 = local read "Numeric 0"() -> (w272:dbl)
                n207 = Tick Count (ms)() -> (millisecond timer value=w274:u32)
                n208 = First Call?() -> (First Call?: T/F=w275:bool)
                n209 = Select(t=w274, s=w275, f=w272) -> (s? t:f=→"Numeric 0":dbl)
              }
              frame #1 {
                n210 = local read "Numeric 0"() -> (w279:dbl)
                n211 = Add(x=500.0, y=w279) -> (x+y=w278:dbl)
                n212 = Tick Count (ms)() -> (millisecond timer value=w277:u32)
                n213 = Less?(x=w278, y=w277) -> (x < y?=w276:bool)
              }
            }
            n214 = call <vilib>:"WPI_RobotDriveRefNum Registry Get.vi"("refnum name"="Left and Right Motors") -> ("RobotDriveDevRef"=w270:T9)  [unwired: 1 in, 9 out]
            n215 = call <vilib>:"WPI_RobotDriveArcadeDrive_Standard(NoSaturation).vi"("Y axis value"=-1.0 ("X axis value"), "X axis value"=0.0, "RobotDriveDevRef"=w270) -> ("Motor Values"=w268:dbl[])  [unwired: 1 in, 7 out]
            n216 = call <vilib>:"SD Write Numeric Array.vi"("Numeric Array"=w268, "Name"="RobotDrive Motors") -> ()  [unwired: 8 in, 2 out]
          }
        }
        frame #1 {
          n217 = while {
            stop <- w281 stop-if-true
            n218 = stacked-sequence {
              tunnel: [_ w292] -> w281
              frame #0 {
                n219 = local read "Numeric 0"() -> (w289:dbl)
                n220 = Tick Count (ms)() -> (millisecond timer value=w290:u32)
                n221 = First Call?() -> (First Call?: T/F=w291:bool)
                n222 = Select(t=w290, s=w291, f=w289) -> (s? t:f=w288:dbl)
                n223 = local write "Numeric 0"(w288) -> ()
              }
              frame #1 {
                n224 = local read "Numeric 0"() -> (w295:dbl)
                n225 = Add(x=250.0, y=w295) -> (x+y=w294:dbl)
                n226 = Tick Count (ms)() -> (millisecond timer value=w293:u32)
                n227 = Less?(x=w294, y=w293) -> (x < y?=w292:bool)
              }
            }
            n228 = call <vilib>:"WPI_RobotDriveRefNum Registry Get.vi"("refnum name"="Left and Right Motors") -> ("RobotDriveDevRef"=w283:T9)  [unwired: 1 in, 9 out]
            n229 = call <vilib>:"WPI_RobotDriveArcadeDrive_Standard(NoSaturation).vi"("Y axis value"=0.0 ("X axis value"), "X axis value"=1.0, "RobotDriveDevRef"=w283) -> ("Motor Values"=w285:dbl[])  [unwired: 1 in, 7 out]
            n230 = call <vilib>:"SD Write Numeric Array.vi"("Numeric Array"=w285, "Name"="RobotDrive Motors") -> ()  [unwired: 8 in, 2 out]
          }
        }
        frame #2 {
          n231 = while {
            stop <- w396 stop-if-true
            # "Ordered Position Array"
            # "DistanceArray"
            n232 = global read "Robot Global Data.vi" "Target Info"() -> (w412:T17)
            n233 = Array To Cluster(array=w412) -> (cluster=w411:T18)
            n234 = Unbundle By Name(w411) -> ("Target Info[0]"=w365:T19, "Target Info[1]"=w407:T19, "Target Info[2]"=w406:T19, "Target Info[3]"=w405:T19)
            n235 = Unbundle By Name(w365) -> ("Center Position"=w364:cluster{"X":dbl, "Y":dbl}, "Distance (ft)"=w384:dbl)  [unwired: 1 out]
            n236 = Unbundle By Name(w407) -> ("Center Position"=w410:cluster{"X":dbl, "Y":dbl}, "Distance (ft)"=w383:dbl)  [unwired: 1 out]
            n237 = Unbundle By Name(w406) -> ("Center Position"=w409:cluster{"X":dbl, "Y":dbl}, "Distance (ft)"=w382:dbl)  [unwired: 1 out]
            n238 = Unbundle By Name(w405) -> ("Center Position"=w408:cluster{"X":dbl, "Y":dbl}, "Distance (ft)"=w381:dbl)  [unwired: 1 out]
            n239 = Unbundle By Name(w364) -> ("X"=w369:dbl)  [unwired: 1 out]
            n240 = Unbundle By Name(w410) -> ("X"=w370:dbl)  [unwired: 1 out]
            n241 = Unbundle By Name(w409) -> ("X"=w375:dbl)  [unwired: 1 out]
            n242 = Unbundle By Name(w408) -> ("X"=w373:dbl)  [unwired: 1 out]
            n243 = Equal To 0?(x=w383) -> (x = 0?=w404:bool)
            n244 = Equal To 0?(x=w382) -> (x = 0?=w403:bool)
            n245 = Equal To 0?(x=w381) -> (x = 0?=w402:bool)
            n246 = Initialize Array(0.0 ("element"), 1 ("dimension size")) -> (w385:dbl[])
            n247 = Absolute Value(x=w369) -> (abs(x)=w368:dbl)
            n248 = Build Array (concatenate)(w385, w384, w383, w382, w381) -> (w366:dbl[])
            n249 = Select(t=1.0, s=w404, f=w370) -> (s? t:f=w371:dbl)
            n250 = Select(t=1.0, s=w403, f=w375) -> (s? t:f=w374:dbl)
            n251 = Select(t=1.0, s=w402, f=w373) -> (s? t:f=w398:dbl)
            n252 = Absolute Value(x=w371) -> (abs(x)=w392:dbl)
            n253 = Absolute Value(x=w374) -> (abs(x)=w391:dbl)
            n254 = Absolute Value(x=w398) -> (abs(x)=w372:dbl)
            n255 = Initialize Array(0.0 ("element"), 1 ("dimension size")) -> (w393:dbl[])
            n256 = Build Array (concatenate)(w393, w368, w392, w391, w372) -> (w388:dbl[])
            n257 = Sort 1D Array(array=w388) -> (sorted array=w367:dbl[])
            n258 = Index Array(array=w367, index=0) -> (element=w389:dbl)
            n259 = Search 1D Array(1D array=w388, element=w389) -> (index of element=w380:i32)  [unwired: 1 in]
            n260 = Index Array(array=w366, index=w380) -> (element=w378:dbl)
            n261 = Subtract(x=w378, y="Sweet Spot") -> (x-y=w377:dbl)
            n262 = Not Equal To 0?(x=w377) -> (x != 0?=w376:bool)
            n263 = case shown="True" w376 {
              tunnel: [1.0 ("output") w421] -> w397
              tunnel: w377 -> [_ w422]
              frame False {
                n264 = call <vilib>:"WPI_RobotDriveRefNum Registry Get.vi"("refnum name"="Left and Right Motors") -> ("RobotDriveDevRef"=w418:T9)  [unwired: 1 in, 9 out]
                n265 = call <vilib>:"WPI_RobotDriveArcadeDrive_Standard(NoSaturation).vi"("Y axis value"=0.0, "X axis value"=0.0, "RobotDriveDevRef"=w418) -> ("Motor Values"=w416:dbl[])  [unwired: 1 in, 7 out]
                n266 = call <vilib>:"SD Write Numeric Array.vi"("Numeric Array"=w416, "Name"="RobotDrive Motors") -> ()  [unwired: 8 in, 2 out]
              }
              frame True {
                n267 = call-poly <vilib>:"PID.vi"("PID gains"="PID gains", "process variable"=w422, "setpoint"=0.0 ("process variable")) -> ("output"=w423:dbl)  [unwired: 7 in, 1 out]
                n268 = In Range and Coerce(upper limit=0.01, x=w423, lower limit=-0.01) -> (In Range?=w425:bool)  [unwired: 1 out]
                n269 = call <vilib>:"WPI_RobotDriveRefNum Registry Get.vi"("refnum name"="Left and Right Motors") -> ("RobotDriveDevRef"=w430:T9)  [unwired: 1 in, 9 out]
                n270 = Select(t=0.0, s=w425, f=w423) -> (s? t:f=w421:dbl)
                n271 = call <vilib>:"WPI_RobotDriveArcadeDrive_Standard(NoSaturation).vi"("Y axis value"=w421, "X axis value"=0.0, "RobotDriveDevRef"=w430) -> ("Motor Values"=w429:dbl[])  [unwired: 1 in, 7 out]
                n272 = call <vilib>:"SD Write Numeric Array.vi"("Numeric Array"=w429, "Name"="RobotDrive Motors") -> ()  [unwired: 8 in, 2 out]
              }
            }
            n273 = Equal To 0?(x=w397) -> (x = 0?=w396:bool)
          }
          n274 = while {
            stop <- w324 stop-if-true
            n275 = global read "Robot Global Data.vi" "Target Info"() -> (w342:T17)
            n276 = Array To Cluster(array=w342) -> (cluster=w341:T18)
            n277 = Unbundle By Name(w341) -> ("Target Info[0]"=w340:T19, "Target Info[1]"=w335:T19, "Target Info[2]"=w334:T19, "Target Info[3]"=w333:T19)
            n278 = Unbundle By Name(w340) -> ("Center Position"=w339:cluster{"X":dbl, "Y":dbl})  [unwired: 2 out]
            n279 = Unbundle By Name(w335) -> ("Center Position"=w338:cluster{"X":dbl, "Y":dbl}, "Distance (ft)"=w302:dbl)  [unwired: 1 out]
            n280 = Unbundle By Name(w334) -> ("Center Position"=w337:cluster{"X":dbl, "Y":dbl}, "Distance (ft)"=w304:dbl)  [unwired: 1 out]
            n281 = Unbundle By Name(w333) -> ("Center Position"=w336:cluster{"X":dbl, "Y":dbl}, "Distance (ft)"=w306:dbl)  [unwired: 1 out]
            n282 = Unbundle By Name(w339) -> ("X"=w297:dbl)  [unwired: 1 out]
            n283 = Unbundle By Name(w338) -> ("X"=w301:dbl)  [unwired: 1 out]
            n284 = Unbundle By Name(w337) -> ("X"=w303:dbl)  [unwired: 1 out]
            n285 = Unbundle By Name(w336) -> ("X"=w305:dbl)  [unwired: 1 out]
            n286 = Equal To 0?(x=w302) -> (x = 0?=w332:bool)
            n287 = Equal To 0?(x=w304) -> (x = 0?=w331:bool)
            n288 = Equal To 0?(x=w306) -> (x = 0?=w330:bool)
            n289 = Initialize Array(0.0 ("element"), 1 ("dimension size")) -> (w308:dbl[])
            n290 = Select(t=1.0, s=w332, f=w301) -> (s? t:f=w313:dbl)
            n291 = Select(t=1.0, s=w331, f=w303) -> (s? t:f=w312:dbl)
            n292 = Select(t=1.0, s=w330, f=w305) -> (s? t:f=w326:dbl)
            n293 = Build Array (concatenate)(w308, w297, w301, w303, w305) -> (w298:dbl[])
            n294 = Absolute Value(x=w313) -> (abs(x)=w319:dbl)
            n295 = Absolute Value(x=w312) -> (abs(x)=w318:dbl)
            n296 = Absolute Value(x=w326) -> (abs(x)=w311:dbl)
            n297 = Absolute Value(x=w297) -> (abs(x)=w320:dbl)
            n298 = Initialize Array(0.0 ("element"), 1 ("dimension size")) -> (w321:dbl[])
            n299 = Build Array (concatenate)(w321, w320, w319, w318, w311) -> (w314:dbl[])
            n300 = Sort 1D Array(array=w314) -> (sorted array=w317:dbl[])
            n301 = Index Array(array=w317, index=0) -> (element=w315:dbl)
            n302 = Search 1D Array(1D array=w314, element=w315) -> (index of element=w307:i32)  [unwired: 1 in]
            n303 = Index Array(array=w298, index=w307) -> (element=w299:dbl)
            n304 = Not Equal To 0?(x=w299) -> (x != 0?=w300:bool)
            n305 = case shown="True" w300 {
              tunnel: [1.0 ("output") w352] -> w325
              tunnel: w299 -> [_ w351]
              frame False {
                n306 = call <vilib>:"WPI_RobotDriveRefNum Registry Get.vi"("refnum name"="Left and Right Motors") -> ("RobotDriveDevRef"=w348:T9)  [unwired: 1 in, 9 out]
                n307 = call <vilib>:"WPI_RobotDriveArcadeDrive_Standard(NoSaturation).vi"("Y axis value"=0.0, "X axis value"=0.0, "RobotDriveDevRef"=w348) -> ("Motor Values"=w346:dbl[])  [unwired: 1 in, 7 out]
                n308 = call <vilib>:"SD Write Numeric Array.vi"("Numeric Array"=w346, "Name"="RobotDrive Motors") -> ()  [unwired: 8 in, 2 out]
              }
              frame True {
                n309 = local read "PID gains"() -> (w350:T2)
                n310 = call-poly <vilib>:"PID.vi"("PID gains"=w350, "process variable"=w351, "setpoint"=0.0 ("process variable")) -> ("output"=w353:dbl)  [unwired: 7 in, 1 out]
                n311 = In Range and Coerce(upper limit=0.01, x=w353, lower limit=-0.01) -> (In Range?=w355:bool)  [unwired: 1 out]
                n312 = call <vilib>:"WPI_RobotDriveRefNum Registry Get.vi"("refnum name"="Left and Right Motors") -> ("RobotDriveDevRef"=w361:T9)  [unwired: 1 in, 9 out]
                n313 = Select(t=0.0, s=w355, f=w353) -> (s? t:f=w352:dbl)
                n314 = call <vilib>:"WPI_RobotDriveArcadeDrive_Standard(NoSaturation).vi"("Y axis value"=0.0, "X axis value"=w352, "RobotDriveDevRef"=w361) -> ("Motor Values"=w360:dbl[])  [unwired: 1 in, 7 out]
                n315 = call <vilib>:"SD Write Numeric Array.vi"("Numeric Array"=w360, "Name"="RobotDrive Motors") -> ()  [unwired: 8 in, 2 out]
              }
            }
            n316 = Equal To 0?(x=w325) -> (x = 0?=w324:bool)
          }
        }
        frame #3 {
          n317 = while {
            stop <- w434 stop-if-true
            # "Slow motor will always be slower"
            n318 = stacked-sequence {
              tunnel: [_ w456] -> w434
              frame #0 {
                n319 = local read "Numeric 0"() -> (w453:dbl)
                n320 = Tick Count (ms)() -> (millisecond timer value=w454:u32)
                n321 = First Call?() -> (First Call?: T/F=w455:bool)
                n322 = Select(t=w454, s=w455, f=w453) -> (s? t:f=w452:dbl)
                n323 = local write "Numeric 0"(w452) -> ()
              }
              frame #1 {
                n324 = local read "Numeric 0"() -> (w459:dbl)
                n325 = Add(x=5000.0, y=w459) -> (x+y=w458:dbl)
                n326 = Tick Count (ms)() -> (millisecond timer value=w457:u32)
                n327 = Less?(x=w458, y=w457) -> (x < y?=w456:bool)
              }
            }
            n328 = call <vilib>:"WPI_JoystickRefNum Registry Get.vi"("refnum name"="Joystick 1") -> ("JoystickDevRef"=w449:T5)  [unwired: 1 in, 9 out]
            n329 = call <vilib>:"WPI_JoystickGet.vi"("JoystickDevRef"=w449) -> ("Axes"=w450:T7)  [unwired: 1 in, 5 out]
            n330 = Unbundle By Name(w450) -> ("axis 3 (throttle)"=w451:dbl)
            n331 = Subtract(x=1.0, y=w451) -> (x-y=w445:dbl)
            n332 = call <vilib>:"WPI_MotorControlRefNum Registry Get.vi"("refnum name"="Launch Motor Fast") -> ("error out"=w439:errorcluster, "MotorControlDevRef"=w438:T10)  [unwired: 9 in]
            n333 = In Range and Coerce(upper limit=1.0, x=w445, lower limit=0.0) -> (coerced(x)=w444:dbl)  [unwired: 1 out]
            n334 = Divide(x=w444, y="Fast-Slow Variable") -> (x/y=w441:dbl)
            n335 = call <vilib>:"WPI_MotorControlSetOutput.vi"("error in (no error)"=w439, "Output"=w444, "MotorControlDevRef"=w438) -> ()  [unwired: 6 in, 3 out]
            n336 = call <vilib>:"WPI_MotorControlRefNum Registry Get.vi"("refnum name"="Launch Motor Slow") -> ("error out"=w436:errorcluster, "MotorControlDevRef"=w437:T10)  [unwired: 9 in]
            n337 = call <vilib>:"WPI_MotorControlSetOutput.vi"("error in (no error)"=w436, "Output"=w441, "MotorControlDevRef"=w437) -> ()  [unwired: 6 in, 3 out]
          }
        }
        frame #4 {
          n338 = while {
            stop <- w461 stop-if-true
            n339 = stacked-sequence {
              tunnel: [_ w471] -> w461
              frame #0 {
                n340 = local read "Numeric 0"() -> (w468:dbl)
                n341 = Tick Count (ms)() -> (millisecond timer value=w469:u32)
                n342 = First Call?() -> (First Call?: T/F=w470:bool)
                n343 = Select(t=w469, s=w470, f=w468) -> (s? t:f=w467:dbl)
                n344 = local write "Numeric 0"(w467) -> ()
              }
              frame #1 {
                n345 = local read "Numeric 0"() -> (w474:dbl)
                n346 = Add(x=1000.0, y=w474) -> (x+y=w473:dbl)
                n347 = Tick Count (ms)() -> (millisecond timer value=w472:u32)
                n348 = Less?(x=w473, y=w472) -> (x < y?=w471:bool)
              }
            }
            n349 = Tick Count (ms)() -> (millisecond timer value=w462:u32)
            n350 = First Call?() -> (First Call?: T/F=w466:bool)
            n351 = case shown="False" w466 {
              tunnel: w462 -> [w480 w484]
              tunnel: [w476 WPI_SolenoidValue."Forward" ("Value")] -> w465
              frame False {
                n352 = local read "tick"() -> (w481:dbl)
                n353 = Less Or Equal?(x=w481, y=w480) -> (x <= y?=w477:bool)
                n354 = Select(t=WPI_SolenoidValue."Reverse" ("Value"), s=w477, f=WPI_SolenoidValue."Forward" ("Value")) -> (s? t:f=w476:T8)
              }
              frame True {
                n355 = Add(x=w484, y="wait time") -> (x+y=→"tick":dbl)
              }
            }
            n356 = call <vilib>:"WPI_SolenoidRefNum Registry Get.vi"("refnum name"="Launch Cylinder") -> ("SolenoidDevRef"=w464:T20)  [unwired: 9 in, 1 out]
            n357 = call-poly <vilib>:"WPI_SolenoidSet.vi"("Value"=w465, "SolenoidDevRef"=w464) -> ()  [unwired: 8 in, 2 out]
          }
        }
        frame #5 {
          n358 = while {
            stop <- w486 stop-if-true
            n359 = stacked-sequence {
              tunnel: [_ w497] -> w486
              frame #0 {
                n360 = local read "Numeric 0"() -> (w493:dbl)
                n361 = Tick Count (ms)() -> (millisecond timer value=w494:u32)
                n362 = First Call?() -> (First Call?: T/F=w495:bool)
                n363 = Select(t=w494, s=w495, f=w493) -> (s? t:f=w492:dbl)
                n364 = local write "Numeric 0"(w492) -> ()
              }
              frame #1 {
                n365 = local read "Numeric 0"() -> (w496:dbl)
                n366 = Add(x=1000.0, y=w496) -> (x+y=w499:dbl)
                n367 = Tick Count (ms)() -> (millisecond timer value=w498:u32)
                n368 = Less?(x=w499, y=w498) -> (x < y?=w497:bool)
              }
            }
            n369 = Tick Count (ms)() -> (millisecond timer value=w487:u32)
            n370 = First Call?() -> (First Call?: T/F=w491:bool)
            n371 = case shown="True" w491 {
              tunnel: w487 -> [w506 w510]
              tunnel: [w502 WPI_SolenoidValue."Forward" ("Value")] -> w490
              frame False {
                n372 = local read "tick"() -> (w501:dbl)
                n373 = Less Or Equal?(x=w501, y=w506) -> (x <= y?=w503:bool)
                n374 = Select(t=WPI_SolenoidValue."Reverse" ("Value"), s=w503, f=WPI_SolenoidValue."Forward" ("Value")) -> (s? t:f=w502:T8)
              }
              frame True {
                n375 = local read "wait time"() -> (w508:dbl)
                n376 = Add(x=w510, y=w508) -> (x+y=w507:dbl)
                n377 = local write "tick"(w507) -> ()
              }
            }
            n378 = call <vilib>:"WPI_SolenoidRefNum Registry Get.vi"("refnum name"="Launch Cylinder") -> ("SolenoidDevRef"=w489:T20)  [unwired: 9 in, 1 out]
            n379 = call-poly <vilib>:"WPI_SolenoidSet.vi"("Value"=w490, "SolenoidDevRef"=w489) -> ()  [unwired: 8 in, 2 out]
          }
        }
      }
    }
    frame "Far Left" {
      n380 = stacked-sequence {
        frame #0 {
          n381 = while {
            stop <- w511 stop-if-true
            n382 = stacked-sequence {
              tunnel: [_ w522] -> w511
              frame #0 {
                n383 = local read "Numeric 0"() -> (w519:dbl)
                n384 = Tick Count (ms)() -> (millisecond timer value=w520:u32)
                n385 = First Call?() -> (First Call?: T/F=w521:bool)
                n386 = Select(t=w520, s=w521, f=w519) -> (s? t:f=w518:dbl)
                n387 = local write "Numeric 0"(w518) -> ()
              }
              frame #1 {
                n388 = local read "Numeric 0"() -> (w525:dbl)
                n389 = Add(x=500.0, y=w525) -> (x+y=w524:dbl)
                n390 = Tick Count (ms)() -> (millisecond timer value=w523:u32)
                n391 = Less?(x=w524, y=w523) -> (x < y?=w522:bool)
              }
            }
            n392 = call <vilib>:"WPI_RobotDriveRefNum Registry Get.vi"("refnum name"="Left and Right Motors") -> ("RobotDriveDevRef"=w516:T9)  [unwired: 1 in, 9 out]
            n393 = call <vilib>:"WPI_RobotDriveArcadeDrive_Standard(NoSaturation).vi"("Y axis value"=-1.0 ("X axis value"), "X axis value"=0.0, "RobotDriveDevRef"=w516) -> ("Motor Values"=w514:dbl[])  [unwired: 1 in, 7 out]
            n394 = call <vilib>:"SD Write Numeric Array.vi"("Numeric Array"=w514, "Name"="RobotDrive Motors") -> ()  [unwired: 8 in, 2 out]
          }
        }
        frame #1 {
          n395 = while {
            stop <- w527 stop-if-true
            n396 = stacked-sequence {
              tunnel: [_ w538] -> w527
              frame #0 {
                n397 = local read "Numeric 0"() -> (w535:dbl)
                n398 = Tick Count (ms)() -> (millisecond timer value=w536:u32)
                n399 = First Call?() -> (First Call?: T/F=w537:bool)
                n400 = Select(t=w536, s=w537, f=w535) -> (s? t:f=w534:dbl)
                n401 = local write "Numeric 0"(w534) -> ()
              }
              frame #1 {
                n402 = local read "Numeric 0"() -> (w541:dbl)
                n403 = Add(x=250.0, y=w541) -> (x+y=w540:dbl)
                n404 = Tick Count (ms)() -> (millisecond timer value=w539:u32)
                n405 = Less?(x=w540, y=w539) -> (x < y?=w538:bool)
              }
            }
            n406 = call <vilib>:"WPI_RobotDriveRefNum Registry Get.vi"("refnum name"="Left and Right Motors") -> ("RobotDriveDevRef"=w529:T9)  [unwired: 1 in, 9 out]
            n407 = call <vilib>:"WPI_RobotDriveArcadeDrive_Standard(NoSaturation).vi"("Y axis value"=0.0 ("X axis value"), "X axis value"=-1.0, "RobotDriveDevRef"=w529) -> ("Motor Values"=w531:dbl[])  [unwired: 1 in, 7 out]
            n408 = call <vilib>:"SD Write Numeric Array.vi"("Numeric Array"=w531, "Name"="RobotDrive Motors") -> ()  [unwired: 8 in, 2 out]
          }
        }
        frame #2 {
          n409 = while {
            stop <- w570 stop-if-true
            n410 = global read "Robot Global Data.vi" "Target Info"() -> (w588:T17)
            n411 = Array To Cluster(array=w588) -> (cluster=w587:T18)
            n412 = Unbundle By Name(w587) -> ("Target Info[0]"=w586:T19, "Target Info[1]"=w581:T19, "Target Info[2]"=w580:T19, "Target Info[3]"=w579:T19)
            n413 = Unbundle By Name(w586) -> ("Center Position"=w585:cluster{"X":dbl, "Y":dbl})  [unwired: 2 out]
            n414 = Unbundle By Name(w581) -> ("Center Position"=w584:cluster{"X":dbl, "Y":dbl}, "Distance (ft)"=w547:dbl)  [unwired: 1 out]
            n415 = Unbundle By Name(w580) -> ("Center Position"=w583:cluster{"X":dbl, "Y":dbl}, "Distance (ft)"=w549:dbl)  [unwired: 1 out]
            n416 = Unbundle By Name(w579) -> ("Center Position"=w582:cluster{"X":dbl, "Y":dbl}, "Distance (ft)"=w551:dbl)  [unwired: 1 out]
            n417 = Unbundle By Name(w585) -> ("X"=w545:dbl)  [unwired: 1 out]
            n418 = Unbundle By Name(w584) -> ("X"=w546:dbl)  [unwired: 1 out]
            n419 = Unbundle By Name(w583) -> ("X"=w548:dbl)  [unwired: 1 out]
            n420 = Unbundle By Name(w582) -> ("X"=w550:dbl)  [unwired: 1 out]
            n421 = Equal To 0?(x=w547) -> (x = 0?=w578:bool)
            n422 = Equal To 0?(x=w549) -> (x = 0?=w577:bool)
            n423 = Equal To 0?(x=w551) -> (x = 0?=w576:bool)
            n424 = Initialize Array(0.0 ("element"), 1 ("dimension size")) -> (w554:dbl[])
            n425 = Select(t=1.0, s=w578, f=w546) -> (s? t:f=w559:dbl)
            n426 = Select(t=1.0, s=w577, f=w548) -> (s? t:f=w558:dbl)
            n427 = Select(t=1.0, s=w576, f=w550) -> (s? t:f=w572:dbl)
            n428 = Build Array (concatenate)(w554, w545, w546, w548, w550) -> (w553:dbl[])
            n429 = Absolute Value(x=w545) -> (abs(x)=w566:dbl)
            n430 = Absolute Value(x=w559) -> (abs(x)=w565:dbl)
            n431 = Absolute Value(x=w558) -> (abs(x)=w564:dbl)
            n432 = Absolute Value(x=w572) -> (abs(x)=w557:dbl)
            n433 = Initialize Array(0.0 ("element"), 1 ("dimension size")) -> (w567:dbl[])
            n434 = Build Array (concatenate)(w567, w566, w565, w564, w557) -> (w560:dbl[])
            n435 = Sort 1D Array(array=w560) -> (sorted array=w563:dbl[])
            n436 = Index Array(array=w563, index=0) -> (element=w561:dbl)
            n437 = Search 1D Array(1D array=w560, element=w561) -> (index of element=w552:i32)  [unwired: 1 in]
            n438 = Index Array(array=w553, index=w552) -> (element=w543:dbl)
            n439 = Not Equal To 0?(x=w543) -> (x != 0?=w544:bool)
            n440 = case shown="True" w544 {
              tunnel: [1.0 ("output") w598] -> w571
              tunnel: w543 -> [_ w597]
              frame False {
                n441 = call <vilib>:"WPI_RobotDriveRefNum Registry Get.vi"("refnum name"="Left and Right Motors") -> ("RobotDriveDevRef"=w594:T9)  [unwired: 1 in, 9 out]
                n442 = call <vilib>:"WPI_RobotDriveArcadeDrive_Standard(NoSaturation).vi"("Y axis value"=0.0, "X axis value"=0.0, "RobotDriveDevRef"=w594) -> ("Motor Values"=w592:dbl[])  [unwired: 1 in, 7 out]
                n443 = call <vilib>:"SD Write Numeric Array.vi"("Numeric Array"=w592, "Name"="RobotDrive Motors") -> ()  [unwired: 8 in, 2 out]
              }
              frame True {
                n444 = local read "PID gains"() -> (w596:T2)
                n445 = call-poly <vilib>:"PID.vi"("PID gains"=w596, "process variable"=w597, "setpoint"=0.0 ("process variable")) -> ("output"=w599:dbl)  [unwired: 7 in, 1 out]
                n446 = In Range and Coerce(upper limit=0.01, x=w599, lower limit=-0.01) -> (In Range?=w601:bool)  [unwired: 1 out]
                n447 = call <vilib>:"WPI_RobotDriveRefNum Registry Get.vi"("refnum name"="Left and Right Motors") -> ("RobotDriveDevRef"=w607:T9)  [unwired: 1 in, 9 out]
                n448 = Select(t=0.0, s=w601, f=w599) -> (s? t:f=w598:dbl)
                n449 = call <vilib>:"WPI_RobotDriveArcadeDrive_Standard(NoSaturation).vi"("Y axis value"=0.0, "X axis value"=w598, "RobotDriveDevRef"=w607) -> ("Motor Values"=w606:dbl[])  [unwired: 1 in, 7 out]
                n450 = call <vilib>:"SD Write Numeric Array.vi"("Numeric Array"=w606, "Name"="RobotDrive Motors") -> ()  [unwired: 8 in, 2 out]
              }
            }
            n451 = Equal To 0?(x=w571) -> (x = 0?=w570:bool)
          }
          n452 = while {
            stop <- w641 stop-if-true
            n453 = global read "Robot Global Data.vi" "Target Info"() -> (w662:T17)
            n454 = Array To Cluster(array=w662) -> (cluster=w661:T18)
            n455 = Unbundle By Name(w661) -> ("Target Info[0]"=w660:T19, "Target Info[1]"=w655:T19, "Target Info[2]"=w654:T19, "Target Info[3]"=w653:T19)
            n456 = Unbundle By Name(w660) -> ("Center Position"=w659:cluster{"X":dbl, "Y":dbl}, "Distance (ft)"=w619:dbl)  [unwired: 1 out]
            n457 = Unbundle By Name(w655) -> ("Center Position"=w658:cluster{"X":dbl, "Y":dbl}, "Distance (ft)"=w618:dbl)  [unwired: 1 out]
            n458 = Unbundle By Name(w654) -> ("Center Position"=w657:cluster{"X":dbl, "Y":dbl}, "Distance (ft)"=w617:dbl)  [unwired: 1 out]
            n459 = Unbundle By Name(w653) -> ("Center Position"=w656:cluster{"X":dbl, "Y":dbl}, "Distance (ft)"=w616:dbl)  [unwired: 1 out]
            n460 = Unbundle By Name(w659) -> ("X"=w627:dbl)  [unwired: 1 out]
            n461 = Unbundle By Name(w658) -> ("X"=w644:dbl)  [unwired: 1 out]
            n462 = Unbundle By Name(w657) -> ("X"=w651:dbl)  [unwired: 1 out]
            n463 = Unbundle By Name(w656) -> ("X"=w652:dbl)  [unwired: 1 out]
            n464 = Equal To 0?(x=w618) -> (x = 0?=w650:bool)
            n465 = Equal To 0?(x=w617) -> (x = 0?=w649:bool)
            n466 = Equal To 0?(x=w616) -> (x = 0?=w648:bool)
            n467 = Initialize Array(0.0 ("element"), 1 ("dimension size")) -> (w620:dbl[])
            n468 = Build Array (concatenate)(w620, w619, w618, w617, w616) -> (w615:dbl[])
            n469 = Select(t=1.0, s=w650, f=w644) -> (s? t:f=w626:dbl)
            n470 = Select(t=1.0, s=w649, f=w651) -> (s? t:f=w625:dbl)
            n471 = Select(t=1.0, s=w648, f=w652) -> (s? t:f=w643:dbl)
            n472 = Absolute Value(x=w627) -> (abs(x)=w637:dbl)
            n473 = Absolute Value(x=w626) -> (abs(x)=w636:dbl)
            n474 = Absolute Value(x=w625) -> (abs(x)=w635:dbl)
            n475 = Absolute Value(x=w643) -> (abs(x)=w624:dbl)
            n476 = Initialize Array(0.0 ("element"), 1 ("dimension size")) -> (w638:dbl[])
            n477 = Initialize Array(0.0 ("element"), 1 ("dimension size")) -> (w628:dbl[])
            n478 = Build Array (concatenate)(w628, w627, w626, w625, w624) -> (w623:dbl[])
            n479 = Build Array (concatenate)(w638, w637, w636, w635, w624) -> (w631:dbl[])
            n480 = Sort 1D Array(array=w631) -> (sorted array=w634:dbl[])
            n481 = Index Array(array=w634, index=0) -> (element=w632:dbl)
            n482 = Search 1D Array(1D array=w631, element=w632) -> (index of element=w614:i32)  [unwired: 1 in]
            n483 = local read "Sweet Spot"() -> (w610:dbl)
            n484 = Index Array(array=w623, index=w614) -> ()  [unwired: 1 out]
            n485 = Index Array(array=w615, index=w614) -> (element=w613:dbl)
            n486 = Subtract(x=w613, y=w610) -> (x-y=w612:dbl)
            n487 = Not Equal To 0?(x=w612) -> (x != 0?=w611:bool)
            n488 = case shown="True" w611 {
              tunnel: [1.0 ("output") w672] -> w642
              tunnel: w612 -> [_ w673]
              frame False {
                n489 = call <vilib>:"WPI_RobotDriveRefNum Registry Get.vi"("refnum name"="Left and Right Motors") -> ("RobotDriveDevRef"=w668:T9)  [unwired: 1 in, 9 out]
                n490 = call <vilib>:"WPI_RobotDriveArcadeDrive_Standard(NoSaturation).vi"("Y axis value"=0.0, "X axis value"=0.0, "RobotDriveDevRef"=w668) -> ("Motor Values"=w666:dbl[])  [unwired: 1 in, 7 out]
                n491 = call <vilib>:"SD Write Numeric Array.vi"("Numeric Array"=w666, "Name"="RobotDrive Motors") -> ()  [unwired: 8 in, 2 out]
              }
              frame True {
                n492 = local read "PID gains"() -> (w670:T2)
                n493 = call-poly <vilib>:"PID.vi"("PID gains"=w670, "process variable"=w673, "setpoint"=0.0 ("process variable")) -> ("output"=w674:dbl)  [unwired: 7 in, 1 out]
                n494 = In Range and Coerce(upper limit=0.01, x=w674, lower limit=-0.01) -> (In Range?=w676:bool)  [unwired: 1 out]
                n495 = call <vilib>:"WPI_RobotDriveRefNum Registry Get.vi"("refnum name"="Left and Right Motors") -> ("RobotDriveDevRef"=w681:T9)  [unwired: 1 in, 9 out]
                n496 = Select(t=0.0, s=w676, f=w674) -> (s? t:f=w672:dbl)
                n497 = call <vilib>:"WPI_RobotDriveArcadeDrive_Standard(NoSaturation).vi"("Y axis value"=w672, "X axis value"=0.0, "RobotDriveDevRef"=w681) -> ("Motor Values"=w680:dbl[])  [unwired: 1 in, 7 out]
                n498 = call <vilib>:"SD Write Numeric Array.vi"("Numeric Array"=w680, "Name"="RobotDrive Motors") -> ()  [unwired: 8 in, 2 out]
              }
            }
            n499 = Equal To 0?(x=w642) -> (x = 0?=w641:bool)
          }
        }
        frame #3 {
          n500 = while {
            stop <- w685 stop-if-true
            # "Slow motor will always be slower"
            n501 = stacked-sequence {
              tunnel: [_ w706] -> w685
              frame #0 {
                n502 = local read "Numeric 0"() -> (w703:dbl)
                n503 = Tick Count (ms)() -> (millisecond timer value=w704:u32)
                n504 = First Call?() -> (First Call?: T/F=w705:bool)
                n505 = Select(t=w704, s=w705, f=w703) -> (s? t:f=w702:dbl)
                n506 = local write "Numeric 0"(w702) -> ()
              }
              frame #1 {
                n507 = local read "Numeric 0"() -> (w709:dbl)
                n508 = Add(x=5000.0, y=w709) -> (x+y=w708:dbl)
                n509 = Tick Count (ms)() -> (millisecond timer value=w707:u32)
                n510 = Less?(x=w708, y=w707) -> (x < y?=w706:bool)
              }
            }
            n511 = call <vilib>:"WPI_JoystickRefNum Registry Get.vi"("refnum name"="Joystick 1") -> ("JoystickDevRef"=w699:T5)  [unwired: 1 in, 9 out]
            n512 = call <vilib>:"WPI_JoystickGet.vi"("JoystickDevRef"=w699) -> ("Axes"=w700:T7)  [unwired: 1 in, 5 out]
            n513 = Unbundle By Name(w700) -> ("axis 3 (throttle)"=w701:dbl)
            n514 = Subtract(x=1.0, y=w701) -> (x-y=w695:dbl)
            n515 = local read "Fast-Slow Variable"() -> (w684:dbl)
            n516 = call <vilib>:"WPI_MotorControlRefNum Registry Get.vi"("refnum name"="Launch Motor Fast") -> ("error out"=w690:errorcluster, "MotorControlDevRef"=w689:T10)  [unwired: 9 in]
            n517 = In Range and Coerce(upper limit=1.0, x=w695, lower limit=0.0) -> (coerced(x)=w694:dbl)  [unwired: 1 out]
            n518 = Divide(x=w694, y=w684) -> (x/y=w692:dbl)
            n519 = call <vilib>:"WPI_MotorControlSetOutput.vi"("error in (no error)"=w690, "Output"=w694, "MotorControlDevRef"=w689) -> ()  [unwired: 6 in, 3 out]
            n520 = call <vilib>:"WPI_MotorControlRefNum Registry Get.vi"("refnum name"="Launch Motor Slow") -> ("error out"=w687:errorcluster, "MotorControlDevRef"=w688:T10)  [unwired: 9 in]
            n521 = call <vilib>:"WPI_MotorControlSetOutput.vi"("error in (no error)"=w687, "Output"=w692, "MotorControlDevRef"=w688) -> ()  [unwired: 6 in, 3 out]
          }
        }
        frame #4 {
          n522 = while {
            stop <- w711 stop-if-true
            n523 = stacked-sequence {
              tunnel: [_ w721] -> w711
              frame #0 {
                n524 = local read "Numeric 0"() -> (w718:dbl)
                n525 = Tick Count (ms)() -> (millisecond timer value=w719:u32)
                n526 = First Call?() -> (First Call?: T/F=w720:bool)
                n527 = Select(t=w719, s=w720, f=w718) -> (s? t:f=w717:dbl)
                n528 = local write "Numeric 0"(w717) -> ()
              }
              frame #1 {
                n529 = local read "Numeric 0"() -> (w724:dbl)
                n530 = Add(x=1000.0, y=w724) -> (x+y=w723:dbl)
                n531 = Tick Count (ms)() -> (millisecond timer value=w722:u32)
                n532 = Less?(x=w723, y=w722) -> (x < y?=w721:bool)
              }
            }
            n533 = Tick Count (ms)() -> (millisecond timer value=w712:u32)
            n534 = First Call?() -> (First Call?: T/F=w716:bool)
            n535 = case shown="False" w716 {
              tunnel: w712 -> [w730 w735]
              tunnel: [w726 WPI_SolenoidValue."Forward" ("Value")] -> w715
              frame False {
                n536 = local read "tick"() -> (w731:dbl)
                n537 = Less Or Equal?(x=w731, y=w730) -> (x <= y?=w727:bool)
                n538 = Select(t=WPI_SolenoidValue."Reverse" ("Value"), s=w727, f=WPI_SolenoidValue."Forward" ("Value")) -> (s? t:f=w726:T8)
              }
              frame True {
                n539 = local read "wait time"() -> (w733:dbl)
                n540 = Add(x=w735, y=w733) -> (x+y=w732:dbl)
                n541 = local write "tick"(w732) -> ()
              }
            }
            n542 = call <vilib>:"WPI_SolenoidRefNum Registry Get.vi"("refnum name"="Launch Cylinder") -> ("SolenoidDevRef"=w714:T20)  [unwired: 9 in, 1 out]
            n543 = call-poly <vilib>:"WPI_SolenoidSet.vi"("Value"=w715, "SolenoidDevRef"=w714) -> ()  [unwired: 8 in, 2 out]
          }
        }
        frame #5 {
          n544 = while {
            stop <- w736 stop-if-true
            n545 = stacked-sequence {
              tunnel: [_ w747] -> w736
              frame #0 {
                n546 = local read "Numeric 0"() -> (w743:dbl)
                n547 = Tick Count (ms)() -> (millisecond timer value=w744:u32)
                n548 = First Call?() -> (First Call?: T/F=w745:bool)
                n549 = Select(t=w744, s=w745, f=w743) -> (s? t:f=w742:dbl)
                n550 = local write "Numeric 0"(w742) -> ()
              }
              frame #1 {
                n551 = local read "Numeric 0"() -> (w746:dbl)
                n552 = Add(x=1000.0, y=w746) -> (x+y=w749:dbl)
                n553 = Tick Count (ms)() -> (millisecond timer value=w748:u32)
                n554 = Less?(x=w749, y=w748) -> (x < y?=w747:bool)
              }
            }
            n555 = Tick Count (ms)() -> (millisecond timer value=w737:u32)
            n556 = First Call?() -> (First Call?: T/F=w741:bool)
            n557 = case shown="True" w741 {
              tunnel: w737 -> [w756 w760]
              tunnel: [w752 WPI_SolenoidValue."Forward" ("Value")] -> w740
              frame False {
                n558 = local read "tick"() -> (w751:dbl)
                n559 = Less Or Equal?(x=w751, y=w756) -> (x <= y?=w753:bool)
                n560 = Select(t=WPI_SolenoidValue."Reverse" ("Value"), s=w753, f=WPI_SolenoidValue."Forward" ("Value")) -> (s? t:f=w752:T8)
              }
              frame True {
                n561 = local read "wait time"() -> (w758:dbl)
                n562 = Add(x=w760, y=w758) -> (x+y=w757:dbl)
                n563 = local write "tick"(w757) -> ()
              }
            }
            n564 = call <vilib>:"WPI_SolenoidRefNum Registry Get.vi"("refnum name"="Launch Cylinder") -> ("SolenoidDevRef"=w739:T20)  [unwired: 9 in, 1 out]
            n565 = call-poly <vilib>:"WPI_SolenoidSet.vi"("Value"=w740, "SolenoidDevRef"=w739) -> ()  [unwired: 8 in, 2 out]
          }
        }
        frame #6 {
          n566 = while {
            stop <- w761 stop-if-true
            n567 = stacked-sequence {
              tunnel: [_ w772] -> w761
              frame #0 {
                n568 = local read "Numeric 0"() -> (w768:dbl)
                n569 = Tick Count (ms)() -> (millisecond timer value=w769:u32)
                n570 = First Call?() -> (First Call?: T/F=w770:bool)
                n571 = Select(t=w769, s=w770, f=w768) -> (s? t:f=w767:dbl)
                n572 = local write "Numeric 0"(w767) -> ()
              }
              frame #1 {
                n573 = local read "Numeric 0"() -> (w771:dbl)
                n574 = Add(x=1000.0, y=w771) -> (x+y=w774:dbl)
                n575 = Tick Count (ms)() -> (millisecond timer value=w773:u32)
                n576 = Less?(x=w774, y=w773) -> (x < y?=w772:bool)
              }
            }
            n577 = Tick Count (ms)() -> (millisecond timer value=w762:u32)
            n578 = First Call?() -> (First Call?: T/F=w766:bool)
            n579 = case shown="True" w766 {
              tunnel: w762 -> [w781 w785]
              tunnel: [w777 WPI_SolenoidValue."Forward" ("Value")] -> w765
              frame False {
                n580 = local read "tick"() -> (w776:dbl)
                n581 = Less Or Equal?(x=w776, y=w781) -> (x <= y?=w778:bool)
                n582 = Select(t=WPI_SolenoidValue."Reverse" ("Value"), s=w778, f=WPI_SolenoidValue."Forward" ("Value")) -> (s? t:f=w777:T8)
              }
              frame True {
                n583 = local read "wait time"() -> (w783:dbl)
                n584 = Add(x=w785, y=w783) -> (x+y=w782:dbl)
                n585 = local write "tick"(w782) -> ()
              }
            }
            n586 = call <vilib>:"WPI_SolenoidRefNum Registry Get.vi"("refnum name"="Launch Cylinder") -> ("SolenoidDevRef"=w764:T20)  [unwired: 9 in, 1 out]
            n587 = call-poly <vilib>:"WPI_SolenoidSet.vi"("Value"=w765, "SolenoidDevRef"=w764) -> ()  [unwired: 8 in, 2 out]
          }
        }
      }
    }
    frame "Far Right" {
      n588 = stacked-sequence {
        frame #0 {
          n589 = while {
            stop <- w786 stop-if-true
            n590 = stacked-sequence {
              tunnel: [_ w798] -> w786
              frame #0 {
                n591 = local read "Numeric 0"() -> (w794:dbl)
                n592 = Tick Count (ms)() -> (millisecond timer value=w795:u32)
                n593 = First Call?() -> (First Call?: T/F=w796:bool)
                n594 = Select(t=w795, s=w796, f=w794) -> (s? t:f=w793:dbl)
                n595 = local write "Numeric 0"(w793) -> ()
              }
              frame #1 {
                n596 = local read "Numeric 0"() -> (w797:dbl)
                n597 = Add(x=500.0, y=w797) -> (x+y=w800:dbl)
                n598 = Tick Count (ms)() -> (millisecond timer value=w799:u32)
                n599 = Less?(x=w800, y=w799) -> (x < y?=w798:bool)
              }
            }
            n600 = call <vilib>:"WPI_RobotDriveRefNum Registry Get.vi"("refnum name"="Left and Right Motors") -> ("RobotDriveDevRef"=w791:T9)  [unwired: 1 in, 9 out]
            n601 = call <vilib>:"WPI_RobotDriveArcadeDrive_Standard(NoSaturation).vi"("Y axis value"=-1.0 ("X axis value"), "X axis value"=0.0, "RobotDriveDevRef"=w791) -> ("Motor Values"=w789:dbl[])  [unwired: 1 in, 7 out]
            n602 = call <vilib>:"SD Write Numeric Array.vi"("Numeric Array"=w789, "Name"="RobotDrive Motors") -> ()  [unwired: 8 in, 2 out]
          }
        }
        frame #1 {
          n603 = while {
            stop <- w802 stop-if-true
            n604 = stacked-sequence {
              tunnel: [_ w814] -> w802
              frame #0 {
                n605 = local read "Numeric 0"() -> (w810:dbl)
                n606 = Tick Count (ms)() -> (millisecond timer value=w811:u32)
                n607 = First Call?() -> (First Call?: T/F=w812:bool)
                n608 = Select(t=w811, s=w812, f=w810) -> (s? t:f=w809:dbl)
                n609 = local write "Numeric 0"(w809) -> ()
              }
              frame #1 {
                n610 = local read "Numeric 0"() -> (w813:dbl)
                n611 = Add(x=250.0, y=w813) -> (x+y=w816:dbl)
                n612 = Tick Count (ms)() -> (millisecond timer value=w815:u32)
                n613 = Less?(x=w816, y=w815) -> (x < y?=w814:bool)
              }
            }
            n614 = call <vilib>:"WPI_RobotDriveRefNum Registry Get.vi"("refnum name"="Left and Right Motors") -> ("RobotDriveDevRef"=w804:T9)  [unwired: 1 in, 9 out]
            n615 = call <vilib>:"WPI_RobotDriveArcadeDrive_Standard(NoSaturation).vi"("Y axis value"=0.0 ("X axis value"), "X axis value"=1.0, "RobotDriveDevRef"=w804) -> ("Motor Values"=w806:dbl[])  [unwired: 1 in, 7 out]
            n616 = call <vilib>:"SD Write Numeric Array.vi"("Numeric Array"=w806, "Name"="RobotDrive Motors") -> ()  [unwired: 8 in, 2 out]
          }
        }
        frame #2 {
          n617 = while {
            stop <- w845 stop-if-true
            n618 = global read "Robot Global Data.vi" "Target Info"() -> (w863:T17)
            n619 = Array To Cluster(array=w863) -> (cluster=w862:T18)
            n620 = Unbundle By Name(w862) -> ("Target Info[0]"=w861:T19, "Target Info[1]"=w856:T19, "Target Info[2]"=w855:T19, "Target Info[3]"=w854:T19)
            n621 = Unbundle By Name(w861) -> ("Center Position"=w860:cluster{"X":dbl, "Y":dbl})  [unwired: 2 out]
            n622 = Unbundle By Name(w856) -> ("Center Position"=w859:cluster{"X":dbl, "Y":dbl}, "Distance (ft)"=w822:dbl)  [unwired: 1 out]
            n623 = Unbundle By Name(w855) -> ("Center Position"=w858:cluster{"X":dbl, "Y":dbl}, "Distance (ft)"=w824:dbl)  [unwired: 1 out]
            n624 = Unbundle By Name(w854) -> ("Center Position"=w857:cluster{"X":dbl, "Y":dbl}, "Distance (ft)"=w826:dbl)  [unwired: 1 out]
            n625 = Unbundle By Name(w860) -> ("X"=w820:dbl)  [unwired: 1 out]
            n626 = Unbundle By Name(w859) -> ("X"=w821:dbl)  [unwired: 1 out]
            n627 = Unbundle By Name(w858) -> ("X"=w823:dbl)  [unwired: 1 out]
            n628 = Unbundle By Name(w857) -> ("X"=w825:dbl)  [unwired: 1 out]
            n629 = Equal To 0?(x=w822) -> (x = 0?=w853:bool)
            n630 = Equal To 0?(x=w824) -> (x = 0?=w852:bool)
            n631 = Equal To 0?(x=w826) -> (x = 0?=w851:bool)
            n632 = Initialize Array(0.0 ("element"), 1 ("dimension size")) -> (w829:dbl[])
            n633 = Select(t=1.0, s=w853, f=w821) -> (s? t:f=w834:dbl)
            n634 = Select(t=1.0, s=w852, f=w823) -> (s? t:f=w833:dbl)
            n635 = Select(t=1.0, s=w851, f=w825) -> (s? t:f=w847:dbl)
            n636 = Build Array (concatenate)(w829, w820, w821, w823, w825) -> (w828:dbl[])
            n637 = Absolute Value(x=w820) -> (abs(x)=w841:dbl)
            n638 = Absolute Value(x=w834) -> (abs(x)=w840:dbl)
            n639 = Absolute Value(x=w833) -> (abs(x)=w839:dbl)
            n640 = Absolute Value(x=w847) -> (abs(x)=w832:dbl)
            n641 = Initialize Array(0.0 ("element"), 1 ("dimension size")) -> (w842:dbl[])
            n642 = Build Array (concatenate)(w842, w841, w840, w839, w832) -> (w835:dbl[])
            n643 = Sort 1D Array(array=w835) -> (sorted array=w838:dbl[])
            n644 = Index Array(array=w838, index=0) -> (element=w836:dbl)
            n645 = Search 1D Array(1D array=w835, element=w836) -> (index of element=w827:i32)  [unwired: 1 in]
            n646 = Index Array(array=w828, index=w827) -> (element=w818:dbl)
            n647 = Not Equal To 0?(x=w818) -> (x != 0?=w819:bool)
            n648 = case shown="True" w819 {
              tunnel: [1.0 ("output") w873] -> w846
              tunnel: w818 -> [_ w872]
              frame False {
                n649 = call <vilib>:"WPI_RobotDriveRefNum Registry Get.vi"("refnum name"="Left and Right Motors") -> ("RobotDriveDevRef"=w869:T9)  [unwired: 1 in, 9 out]
                n650 = call <vilib>:"WPI_RobotDriveArcadeDrive_Standard(NoSaturation).vi"("Y axis value"=0.0, "X axis value"=0.0, "RobotDriveDevRef"=w869) -> ("Motor Values"=w867:dbl[])  [unwired: 1 in, 7 out]
                n651 = call <vilib>:"SD Write Numeric Array.vi"("Numeric Array"=w867, "Name"="RobotDrive Motors") -> ()  [unwired: 8 in, 2 out]
              }
              frame True {
                n652 = local read "PID gains"() -> (w871:T2)
                n653 = call-poly <vilib>:"PID.vi"("PID gains"=w871, "process variable"=w872, "setpoint"=0.0 ("process variable")) -> ("output"=w874:dbl)  [unwired: 7 in, 1 out]
                n654 = In Range and Coerce(upper limit=0.01, x=w874, lower limit=-0.01) -> (In Range?=w876:bool)  [unwired: 1 out]
                n655 = call <vilib>:"WPI_RobotDriveRefNum Registry Get.vi"("refnum name"="Left and Right Motors") -> ("RobotDriveDevRef"=w882:T9)  [unwired: 1 in, 9 out]
                n656 = Select(t=0.0, s=w876, f=w874) -> (s? t:f=w873:dbl)
                n657 = call <vilib>:"WPI_RobotDriveArcadeDrive_Standard(NoSaturation).vi"("Y axis value"=0.0, "X axis value"=w873, "RobotDriveDevRef"=w882) -> ("Motor Values"=w881:dbl[])  [unwired: 1 in, 7 out]
                n658 = call <vilib>:"SD Write Numeric Array.vi"("Numeric Array"=w881, "Name"="RobotDrive Motors") -> ()  [unwired: 8 in, 2 out]
              }
            }
            n659 = Equal To 0?(x=w846) -> (x = 0?=w845:bool)
          }
          n660 = while {
            stop <- w916 stop-if-true
            n661 = global read "Robot Global Data.vi" "Target Info"() -> (w937:T17)
            n662 = Array To Cluster(array=w937) -> (cluster=w936:T18)
            n663 = Unbundle By Name(w936) -> ("Target Info[0]"=w935:T19, "Target Info[1]"=w930:T19, "Target Info[2]"=w929:T19, "Target Info[3]"=w928:T19)
            n664 = Unbundle By Name(w935) -> ("Center Position"=w934:cluster{"X":dbl, "Y":dbl}, "Distance (ft)"=w894:dbl)  [unwired: 1 out]
            n665 = Unbundle By Name(w930) -> ("Center Position"=w933:cluster{"X":dbl, "Y":dbl}, "Distance (ft)"=w893:dbl)  [unwired: 1 out]
            n666 = Unbundle By Name(w929) -> ("Center Position"=w932:cluster{"X":dbl, "Y":dbl}, "Distance (ft)"=w892:dbl)  [unwired: 1 out]
            n667 = Unbundle By Name(w928) -> ("Center Position"=w931:cluster{"X":dbl, "Y":dbl}, "Distance (ft)"=w891:dbl)  [unwired: 1 out]
            n668 = Unbundle By Name(w934) -> ("X"=w902:dbl)  [unwired: 1 out]
            n669 = Unbundle By Name(w933) -> ("X"=w919:dbl)  [unwired: 1 out]
            n670 = Unbundle By Name(w932) -> ("X"=w926:dbl)  [unwired: 1 out]
            n671 = Unbundle By Name(w931) -> ("X"=w927:dbl)  [unwired: 1 out]
            n672 = Equal To 0?(x=w893) -> (x = 0?=w925:bool)
            n673 = Equal To 0?(x=w892) -> (x = 0?=w924:bool)
            n674 = Equal To 0?(x=w891) -> (x = 0?=w923:bool)
            n675 = Initialize Array(0.0 ("element"), 1 ("dimension size")) -> (w895:dbl[])
            n676 = Build Array (concatenate)(w895, w894, w893, w892, w891) -> (w890:dbl[])
            n677 = Select(t=1.0, s=w925, f=w919) -> (s? t:f=w901:dbl)
            n678 = Select(t=1.0, s=w924, f=w926) -> (s? t:f=w900:dbl)
            n679 = Select(t=1.0, s=w923, f=w927) -> (s? t:f=w918:dbl)
            n680 = Absolute Value(x=w902) -> (abs(x)=w912:dbl)
            n681 = Absolute Value(x=w901) -> (abs(x)=w911:dbl)
            n682 = Absolute Value(x=w900) -> (abs(x)=w910:dbl)
            n683 = Absolute Value(x=w918) -> (abs(x)=w899:dbl)
            n684 = Initialize Array(0.0 ("element"), 1 ("dimension size")) -> (w913:dbl[])
            n685 = Initialize Array(0.0 ("element"), 1 ("dimension size")) -> (w903:dbl[])
            n686 = Build Array (concatenate)(w903, w902, w901, w900, w899) -> (w898:dbl[])
            n687 = Build Array (concatenate)(w913, w912, w911, w910, w899) -> (w906:dbl[])
            n688 = Sort 1D Array(array=w906) -> (sorted array=w909:dbl[])
            n689 = Index Array(array=w909, index=0) -> (element=w907:dbl)
            n690 = Search 1D Array(1D array=w906, element=w907) -> (index of element=w889:i32)  [unwired: 1 in]
            n691 = local read "Sweet Spot"() -> (w885:dbl)
            n692 = Index Array(array=w898, index=w889) -> ()  [unwired: 1 out]
            n693 = Index Array(array=w890, index=w889) -> (element=w888:dbl)
            n694 = Subtract(x=w888, y=w885) -> (x-y=w887:dbl)
            n695 = Not Equal To 0?(x=w887) -> (x != 0?=w886:bool)
            n696 = case shown="True" w886 {
              tunnel: [1.0 ("output") w947] -> w917
              tunnel: w887 -> [_ w948]
              frame False {
                n697 = call <vilib>:"WPI_RobotDriveRefNum Registry Get.vi"("refnum name"="Left and Right Motors") -> ("RobotDriveDevRef"=w943:T9)  [unwired: 1 in, 9 out]
                n698 = call <vilib>:"WPI_RobotDriveArcadeDrive_Standard(NoSaturation).vi"("Y axis value"=0.0, "X axis value"=0.0, "RobotDriveDevRef"=w943) -> ("Motor Values"=w941:dbl[])  [unwired: 1 in, 7 out]
                n699 = call <vilib>:"SD Write Numeric Array.vi"("Numeric Array"=w941, "Name"="RobotDrive Motors") -> ()  [unwired: 8 in, 2 out]
              }
              frame True {
                n700 = local read "PID gains"() -> (w945:T2)
                n701 = call-poly <vilib>:"PID.vi"("PID gains"=w945, "process variable"=w948, "setpoint"=0.0 ("process variable")) -> ("output"=w949:dbl)  [unwired: 7 in, 1 out]
                n702 = In Range and Coerce(upper limit=0.01, x=w949, lower limit=-0.01) -> (In Range?=w951:bool)  [unwired: 1 out]
                n703 = call <vilib>:"WPI_RobotDriveRefNum Registry Get.vi"("refnum name"="Left and Right Motors") -> ("RobotDriveDevRef"=w956:T9)  [unwired: 1 in, 9 out]
                n704 = Select(t=0.0, s=w951, f=w949) -> (s? t:f=w947:dbl)
                n705 = call <vilib>:"WPI_RobotDriveArcadeDrive_Standard(NoSaturation).vi"("Y axis value"=w947, "X axis value"=0.0, "RobotDriveDevRef"=w956) -> ("Motor Values"=w955:dbl[])  [unwired: 1 in, 7 out]
                n706 = call <vilib>:"SD Write Numeric Array.vi"("Numeric Array"=w955, "Name"="RobotDrive Motors") -> ()  [unwired: 8 in, 2 out]
              }
            }
            n707 = Equal To 0?(x=w917) -> (x = 0?=w916:bool)
          }
        }
        frame #3 {
          n708 = while {
            stop <- w960 stop-if-true
            # "Slow motor will always be slower"
            n709 = stacked-sequence {
              tunnel: [_ w982] -> w960
              frame #0 {
                n710 = local read "Numeric 0"() -> (w978:dbl)
                n711 = Tick Count (ms)() -> (millisecond timer value=w979:u32)
                n712 = First Call?() -> (First Call?: T/F=w980:bool)
                n713 = Select(t=w979, s=w980, f=w978) -> (s? t:f=w977:dbl)
                n714 = local write "Numeric 0"(w977) -> ()
              }
              frame #1 {
                n715 = local read "Numeric 0"() -> (w981:dbl)
                n716 = Add(x=5000.0, y=w981) -> (x+y=w984:dbl)
                n717 = Tick Count (ms)() -> (millisecond timer value=w983:u32)
                n718 = Less?(x=w984, y=w983) -> (x < y?=w982:bool)
              }
            }
            n719 = call <vilib>:"WPI_JoystickRefNum Registry Get.vi"("refnum name"="Joystick 1") -> ("JoystickDevRef"=w974:T5)  [unwired: 1 in, 9 out]
            n720 = call <vilib>:"WPI_JoystickGet.vi"("JoystickDevRef"=w974) -> ("Axes"=w975:T7)  [unwired: 1 in, 5 out]
            n721 = Unbundle By Name(w975) -> ("axis 3 (throttle)"=w976:dbl)
            n722 = Subtract(x=1.0, y=w976) -> (x-y=w970:dbl)
            n723 = local read "Fast-Slow Variable"() -> (w959:dbl)
            n724 = call <vilib>:"WPI_MotorControlRefNum Registry Get.vi"("refnum name"="Launch Motor Fast") -> ("error out"=w965:errorcluster, "MotorControlDevRef"=w964:T10)  [unwired: 9 in]
            n725 = In Range and Coerce(upper limit=1.0, x=w970, lower limit=0.0) -> (coerced(x)=w969:dbl)  [unwired: 1 out]
            n726 = Divide(x=w969, y=w959) -> (x/y=w967:dbl)
            n727 = call <vilib>:"WPI_MotorControlSetOutput.vi"("error in (no error)"=w965, "Output"=w969, "MotorControlDevRef"=w964) -> ()  [unwired: 6 in, 3 out]
            n728 = call <vilib>:"WPI_MotorControlRefNum Registry Get.vi"("refnum name"="Launch Motor Slow") -> ("error out"=w962:errorcluster, "MotorControlDevRef"=w963:T10)  [unwired: 9 in]
            n729 = call <vilib>:"WPI_MotorControlSetOutput.vi"("error in (no error)"=w962, "Output"=w967, "MotorControlDevRef"=w963) -> ()  [unwired: 6 in, 3 out]
          }
        }
        frame #4 {
          n730 = while {
            stop <- w986 stop-if-true
            n731 = stacked-sequence {
              tunnel: [_ w997] -> w986
              frame #0 {
                n732 = local read "Numeric 0"() -> (w993:dbl)
                n733 = Tick Count (ms)() -> (millisecond timer value=w994:u32)
                n734 = First Call?() -> (First Call?: T/F=w995:bool)
                n735 = Select(t=w994, s=w995, f=w993) -> (s? t:f=w992:dbl)
                n736 = local write "Numeric 0"(w992) -> ()
              }
              frame #1 {
                n737 = local read "Numeric 0"() -> (w996:dbl)
                n738 = Add(x=1000.0, y=w996) -> (x+y=w999:dbl)
                n739 = Tick Count (ms)() -> (millisecond timer value=w998:u32)
                n740 = Less?(x=w999, y=w998) -> (x < y?=w997:bool)
              }
            }
            n741 = Tick Count (ms)() -> (millisecond timer value=w987:u32)
            n742 = First Call?() -> (First Call?: T/F=w991:bool)
            n743 = case shown="True" w991 {
              tunnel: w987 -> [w1005 w1010]
              tunnel: [w1001 WPI_SolenoidValue."Forward" ("Value")] -> w990
              frame False {
                n744 = local read "tick"() -> (w1006:dbl)
                n745 = Less Or Equal?(x=w1006, y=w1005) -> (x <= y?=w1002:bool)
                n746 = Select(t=WPI_SolenoidValue."Reverse" ("Value"), s=w1002, f=WPI_SolenoidValue."Forward" ("Value")) -> (s? t:f=w1001:T8)
              }
              frame True {
                n747 = local read "wait time"() -> (w1008:dbl)
                n748 = Add(x=w1010, y=w1008) -> (x+y=w1007:dbl)
                n749 = local write "tick"(w1007) -> ()
              }
            }
            n750 = call <vilib>:"WPI_SolenoidRefNum Registry Get.vi"("refnum name"="Launch Cylinder") -> ("SolenoidDevRef"=w989:T20)  [unwired: 9 in, 1 out]
            n751 = call-poly <vilib>:"WPI_SolenoidSet.vi"("Value"=w990, "SolenoidDevRef"=w989) -> ()  [unwired: 8 in, 2 out]
          }
        }
        frame #5 {
          n752 = while {
            stop <- w1011 stop-if-true
            n753 = stacked-sequence {
              tunnel: [_ w1022] -> w1011
              frame #0 {
                n754 = local read "Numeric 0"() -> (w1018:dbl)
                n755 = Tick Count (ms)() -> (millisecond timer value=w1019:u32)
                n756 = First Call?() -> (First Call?: T/F=w1020:bool)
                n757 = Select(t=w1019, s=w1020, f=w1018) -> (s? t:f=w1017:dbl)
                n758 = local write "Numeric 0"(w1017) -> ()
              }
              frame #1 {
                n759 = local read "Numeric 0"() -> (w1021:dbl)
                n760 = Add(x=1000.0, y=w1021) -> (x+y=w1024:dbl)
                n761 = Tick Count (ms)() -> (millisecond timer value=w1023:u32)
                n762 = Less?(x=w1024, y=w1023) -> (x < y?=w1022:bool)
              }
            }
            n763 = Tick Count (ms)() -> (millisecond timer value=w1012:u32)
            n764 = First Call?() -> (First Call?: T/F=w1016:bool)
            n765 = case shown="False" w1016 {
              tunnel: w1012 -> [w1031 w1035]
              tunnel: [w1027 WPI_SolenoidValue."Forward" ("Value")] -> w1015
              frame False {
                n766 = local read "tick"() -> (w1026:dbl)
                n767 = Less Or Equal?(x=w1026, y=w1031) -> (x <= y?=w1028:bool)
                n768 = Select(t=WPI_SolenoidValue."Reverse" ("Value"), s=w1028, f=WPI_SolenoidValue."Forward" ("Value")) -> (s? t:f=w1027:T8)
              }
              frame True {
                n769 = local read "wait time"() -> (w1033:dbl)
                n770 = Add(x=w1035, y=w1033) -> (x+y=w1032:dbl)
                n771 = local write "tick"(w1032) -> ()
              }
            }
            n772 = call <vilib>:"WPI_SolenoidRefNum Registry Get.vi"("refnum name"="Launch Cylinder") -> ("SolenoidDevRef"=w1014:T20)  [unwired: 9 in, 1 out]
            n773 = call-poly <vilib>:"WPI_SolenoidSet.vi"("Value"=w1015, "SolenoidDevRef"=w1014) -> ()  [unwired: 8 in, 2 out]
          }
        }
        frame #6 {
          n774 = while {
            stop <- w1036 stop-if-true
            n775 = stacked-sequence {
              tunnel: [_ w1047] -> w1036
              frame #0 {
                n776 = local read "Numeric 0"() -> (w1043:dbl)
                n777 = Tick Count (ms)() -> (millisecond timer value=w1044:u32)
                n778 = First Call?() -> (First Call?: T/F=w1045:bool)
                n779 = Select(t=w1044, s=w1045, f=w1043) -> (s? t:f=w1042:dbl)
                n780 = local write "Numeric 0"(w1042) -> ()
              }
              frame #1 {
                n781 = local read "Numeric 0"() -> (w1046:dbl)
                n782 = Add(x=1000.0, y=w1046) -> (x+y=w1049:dbl)
                n783 = Tick Count (ms)() -> (millisecond timer value=w1048:u32)
                n784 = Less?(x=w1049, y=w1048) -> (x < y?=w1047:bool)
              }
            }
            n785 = Tick Count (ms)() -> (millisecond timer value=w1037:u32)
            n786 = First Call?() -> (First Call?: T/F=w1041:bool)
            n787 = case shown="True" w1041 {
              tunnel: w1037 -> [w1056 w1060]
              tunnel: [w1052 WPI_SolenoidValue."Forward" ("Value")] -> w1040
              frame False {
                n788 = local read "tick"() -> (w1051:dbl)
                n789 = Less Or Equal?(x=w1051, y=w1056) -> (x <= y?=w1053:bool)
                n790 = Select(t=WPI_SolenoidValue."Reverse" ("Value"), s=w1053, f=WPI_SolenoidValue."Forward" ("Value")) -> (s? t:f=w1052:T8)
              }
              frame True {
                n791 = local read "wait time"() -> (w1058:dbl)
                n792 = Add(x=w1060, y=w1058) -> (x+y=w1057:dbl)
                n793 = local write "tick"(w1057) -> ()
              }
            }
            n794 = call <vilib>:"WPI_SolenoidRefNum Registry Get.vi"("refnum name"="Launch Cylinder") -> ("SolenoidDevRef"=w1039:T20)  [unwired: 9 in, 1 out]
            n795 = call-poly <vilib>:"WPI_SolenoidSet.vi"("Value"=w1040, "SolenoidDevRef"=w1039) -> ()  [unwired: 8 in, 2 out]
          }
        }
      }
    }
  }
  n796 = disable-structure shown="Disabled" {
    frame Disabled {
      # "This sample code describes robot movements in an array. You can extend it to control other motors\non your robot. You can also use file I/O to move the data to a text file."
      n797 = call <vilib>:"WPI_RobotDriveRefNum Registry Get.vi"("refnum name"="Left and Right Motors") -> ("RobotDriveDevRef"=w1062:T9)  [unwired: 1 in, 9 out]
      n798 = for {
        shift-right: [w1068] -> _
        shift-left: w1062 -> [w1069]
        tunnel: "Array of robot movements" -> [w1064] mode=indexing
        n799 = Unbundle By Name(w1064) -> ("X Joystick Value"=w1067:dbl, "Y Joystick Value"=w1066:dbl, "Delay (sec)"=w1065:dbl)  [unwired: 1 out]
        n800 = call-poly <vilib>:"WPI_RobotDriveArcadeDrive.vi"("Y axis value"=w1066, "X axis value"=w1067, "RobotDriveDevRef"=w1069) -> ("Motor Values"=w1071:dbl[], "RobotDriveDevRef"=w1070:T9)  [unwired: 1 in, 6 out]
        n801 = call <vilib>:"SD Write Numeric Array.vi"("Numeric Array"=w1071, "Name"="RobotDrive Motors") -> ()  [unwired: 8 in, 2 out]
        n802 = call <vilib>:"WPI_RobotDriveDelayAndUpdateSafety.vi"("Delay (s)"=w1065, "RobotDriveDevRef"=w1070) -> ("RobotDriveDevRef 2"=w1068:T9)  [unwired: 8 in, 1 out]
        "Current Movement, for debugging" <- w1064
      }
    }
    frame Enabled {
    }
  }
  n803 = disable-structure shown="Disabled" {
    frame Disabled {
      w1073 = "RobotDrive Motors" ("Name")
      # "This is some simple sample code to drive your robot curving one direction and then the other."
      # "stand still"
      # "turn left for 0.5 second"
      # "turn right for 1 second"
      n804 = call <vilib>:"WPI_RobotDriveRefNum Registry Get.vi"("refnum name"="Left and Right Motors") -> ("RobotDriveDevRef"=w1077:T9)  [unwired: 1 in, 9 out]
      n805 = call-poly <vilib>:"WPI_RobotDriveArcadeDrive.vi"("Y axis value"=0.5 ("X axis value"), "X axis value"=0.25, "RobotDriveDevRef"=w1077) -> ("Motor Values"=w1076:dbl[], "RobotDriveDevRef"=w1084:T9)  [unwired: 1 in, 6 out]
      n806 = call <vilib>:"SD Write Numeric Array.vi"("Numeric Array"=w1076, "Name"=w1073) -> ()  [unwired: 8 in, 2 out]
      n807 = call <vilib>:"WPI_RobotDriveDelayAndUpdateSafety.vi"("Delay (s)"=1.0, "RobotDriveDevRef"=w1084) -> ("RobotDriveDevRef 2"=w1083:T9)  [unwired: 8 in, 1 out]
      n808 = call-poly <vilib>:"WPI_RobotDriveArcadeDrive.vi"("Y axis value"=0.25 ("X axis value"), "X axis value"=0.5, "RobotDriveDevRef"=w1083) -> ("Motor Values"=w1075:dbl[], "RobotDriveDevRef"=w1082:T9)  [unwired: 1 in, 6 out]
      n809 = call <vilib>:"SD Write Numeric Array.vi"("Numeric Array"=w1075, "Name"=w1073) -> ()  [unwired: 8 in, 2 out]
      n810 = call <vilib>:"WPI_RobotDriveDelayAndUpdateSafety.vi"("Delay (s)"=0.5, "RobotDriveDevRef"=w1082) -> ("RobotDriveDevRef 2"=w1081:T9)  [unwired: 8 in, 1 out]
      n811 = call-poly <vilib>:"WPI_RobotDriveArcadeDrive.vi"("Y axis value"=0.0 ("X axis value"), "X axis value"=0.0, "RobotDriveDevRef"=w1081) -> ("Motor Values"=w1074:dbl[])  [unwired: 1 in, 7 out]
      n812 = call <vilib>:"SD Write Numeric Array.vi"("Numeric Array"=w1074, "Name"=w1073) -> ()  [unwired: 8 in, 2 out]
    }
    frame Enabled {
    }
  }
